vi "NI-USB-8452 SPI EEPROM Programmer.vi"() -> ()   [LabVIEW 2015]
doc: "This example shows a more generalized way to use the SPI advanced API to write data. It allows the user to change the following parameters: page size, write delay, the endianness of the address bytes, and the number of bytes in an address.\n\nThe parameters will have the following effects:\n\nTarget Page Size (bytes): This places an additional constraint on the amount of bytes written. The smaller value will be used, and that number of bytes written.\nWrite Delay Between Pages (ms): This will force a mandatory delay after writing bytes to a device.\nData Address Width: This will allow the user to specify the EEPROM Data Address as either 1 or 2 bytes.\nData Address Endianness: This control will change the ordering of the bytes in the EEPROM Data Address, note that this only has an effect if there are 2 bytes in the address.\n\nFor connection information see the NI-845x Hardware and Software manual and the manual for your specific SPI device."
uses:
  <vilib>/ni845x/ni845x.llb/ni845xControl.ctl
  <vilib>/ni845x/ni845x.llb/ni845xSpiScriptControl.ctl
  <vilib>/ni845x/ni845x.llb/NI-845x SPI Script Us Delay.vi
  <vilib>/ni845x/ni845x.llb/NI-845x SPI Script Ms Delay.vi
  <vilib>/ni845x/ni845x.llb/NI-845x SPI Close Script Reference.vi
  <vilib>/LAVA/UI Tools/Dialog/Dialog/Dialog/Dialog__lava_lib_ui_tools.lvclass
  <resource>/objmgr/NI845x.rc
panel:
  in  "Verbose?":bool
  in  "Device Data":T1(tab)
  in  "EEPROM Program Data":string[][](table)
  out "Data Bytes Written":u8[](array[numeric]) format="%x"
  out "Read Data":u8[](array[numeric]) format="%x"
  out "Hex Table":string[][](table)
  out "Bin Table":string[][](table)
  in  "EEPROM Device Type":T2(ring)
  in  "Device Mode":enum16{"SPI", "I2C", "DIO"}(ring)
  in  "CS Idle Level":enum16{"Low (Assert High)", "High (Assert Low)"}(ring)
  in  "CLK Phase (CPHS)":i32(ring) items=["0 (First Edge)", "1 (Second Edge)"]
  in  "CLK Polarity (CPOL)":i32(ring) items=["0 (Idle Low)", "1 (Idle High)"]
  in  "IO Level (V)":i32(ring)=33 items=["3.3V"=33, "2.5V"=25, "1.8V"=18, "1.5V"=15, "1.2V"=12]
  in  "CS/SS":u32
  in  "NI845x Device ID":T3="NI-8452"
  in  "CLK Rate (kHz)":u16=2000
  in  "Config INI Save":bool
  in  "Help":bool
  in  "QUIT":bool
  in  "Data Width":enum16{"8 bits", "16 bits"}(ring)
  in  "Address Width":enum16{"8 bits", "16 bits"}(ring)
  in  "Bit Pattern (Write All)":T4(ring)=enum."0xAA (0b10101010)"
  in  "Data Address Endianness":bool=TRUE
  in  "Page Write Delay (ms)":u8=3
  in  "Target Page Size (bytes)":i32=2 min=2 step=2 format="%04x"
  in  "EEPROM Data Address":u16 format="%04x"
  in  "Number of Bytes (Read)":i16=2048 min=4 step=4 format="%04x"
  in  "WRAL":u8=17 format="%08b"
  in  "ERAL":u8=18 format="%08b"
  in  "EWEN":u8=19 format="%08b"
  in  "READ":u8=6 format="%08b"
  in  "WRITE":u8=5 format="%08b"
  in  "EWDS":u8=16 format="%08b"
  in  "Write ALL Device":bool
  in  "Erase ALL Device":bool
  in  "Read Device":bool
  in  "Program Device":bool
  in  "SPI Script Reference":T5
  # "NI-USB-8452 SPI/I2C EEPROM Programmer\n(for 8, 16, 32, 64-bit Devices)"
  # "NI-8451 Device Configuration"
  # "Slave Device Configuration"
  # "Device Data"
  # "1.0_06012020"
  # "Big Endian"
  # "Little Endian"
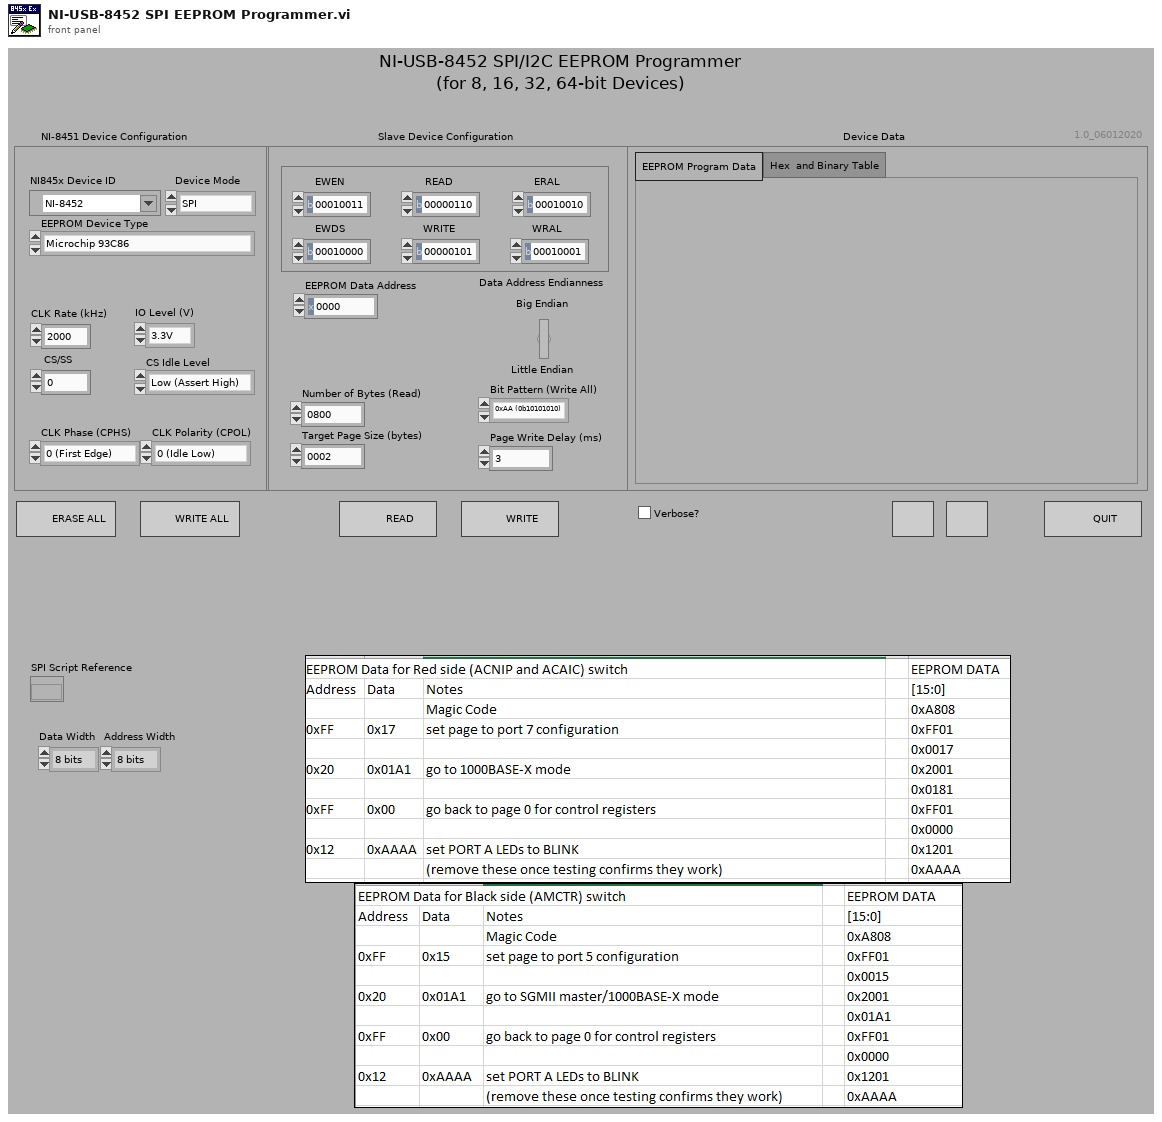
[diagram p1: front panel]
types:
  T1 = enum32{"EEPROM Program Data", "Hex  and Binary Table"}
  T2 = enum16{"Microchip 93C86", "Microchip LC56BT", "Generic EEPROM"}
  T3 = typedef "ni845xControl.ctl" = refnum<k21>
  T4 = enum8{"0xEE (0b11101110)", "0xAA (0b10101010)", "0x55 (0b01010101)", "All ONES", "All ZEROES"}
  T5 = typedef "ni845xSpiScriptControl.ctl" = refnum<k20>
  T6 = enum32{"Invalid", "Standard", "Closed", "Hidden", "Minimized", "Maximized"}
  T7 = enum32{"invalid app kind", "Development System", "Run Time System", "Student Edition", "Embedded LabVIEW", "Evaluation", "Custom"}
  T8 = cluster{"INI Path":path, "SPI Script Reference":T5, "NI845x Device ID":T3, "Device Mode":enum16{"SPI", "I2C", "DIO"}, "EEPROM Device Type":enum16{"Microchip 93C86", "Microchip LC56BT", "Generic EEPROM"}, "Core":cluster{"Current VI Reference":refnum<vi>, "Close Panel on Exit?":bool}, "IO Level (V)":i32, "CS/SS":u32, "CLK Rate (kHz)":u16, "CLK Polarity (CPOL)":i32, "CLK Phase (CPHS)":i32, " Address Width":enum16{"8 bits", "16 bits"}, "Data Width":enum16{"8 bits", "16 bits"}, "EEPROM Data Address":u16, "Number of Bytes (Read)":i16, "Target Page Size (bytes)":i32, "Page Write Delay (ms)":u8, "Array of Write Cluster Information":cluster{"EEPROM Address":u16, "Length":u32, "Data Index":u32}[], "CS Idle Level":enum16{"Low (Assert High)", "High (Assert Low)"}, "script read index":u32, "Bit Pattern (Write All)":enum8{"0xEE (0b11101110)", "0xAA (0b10101010)", "0x55 (0b01010101)", "All ONES", "All ZEROES"}, "READ":u8, "WRITE":u8, "EWEN":u8, "EWDS":u8, "WRAL":u8, "ERAL":u8, "Hex Table":string[][], "Bin Table ":string[][], "EEPROM Program Data ":string[][], "Read Data":u8[], "Data Bytes Written":u8[], "Data Address Endianness":bool, "Verbose?":bool}
  T9 = cluster{"Current VI Reference":refnum<vi>, "Close Panel on Exit?":bool}
  T10 = cluster{"EEPROM Address":u16, "Length":u32, "Data Index":u32}[]
  T11 = typedef "imagedata.ctl" = cluster{"image type":i32, "image depth":i32, "image":u8[], "mask":u8[], "colors":u32[], "Rectangle":cluster{"left":i16, "top":i16, "right":i16, "bottom":i16}}
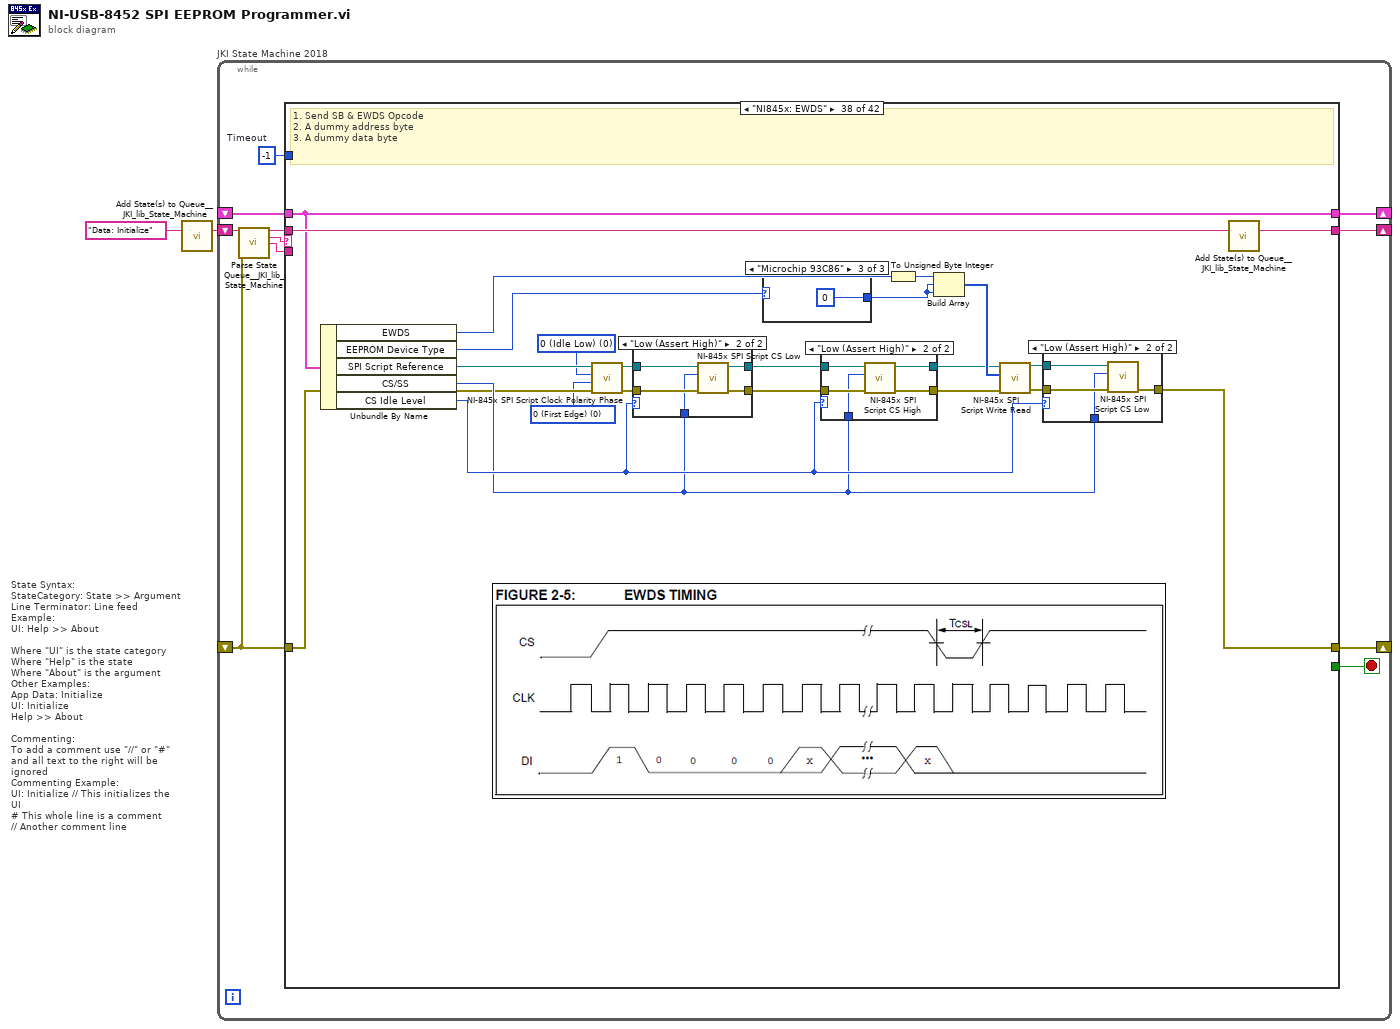
[diagram p0: block diagram]
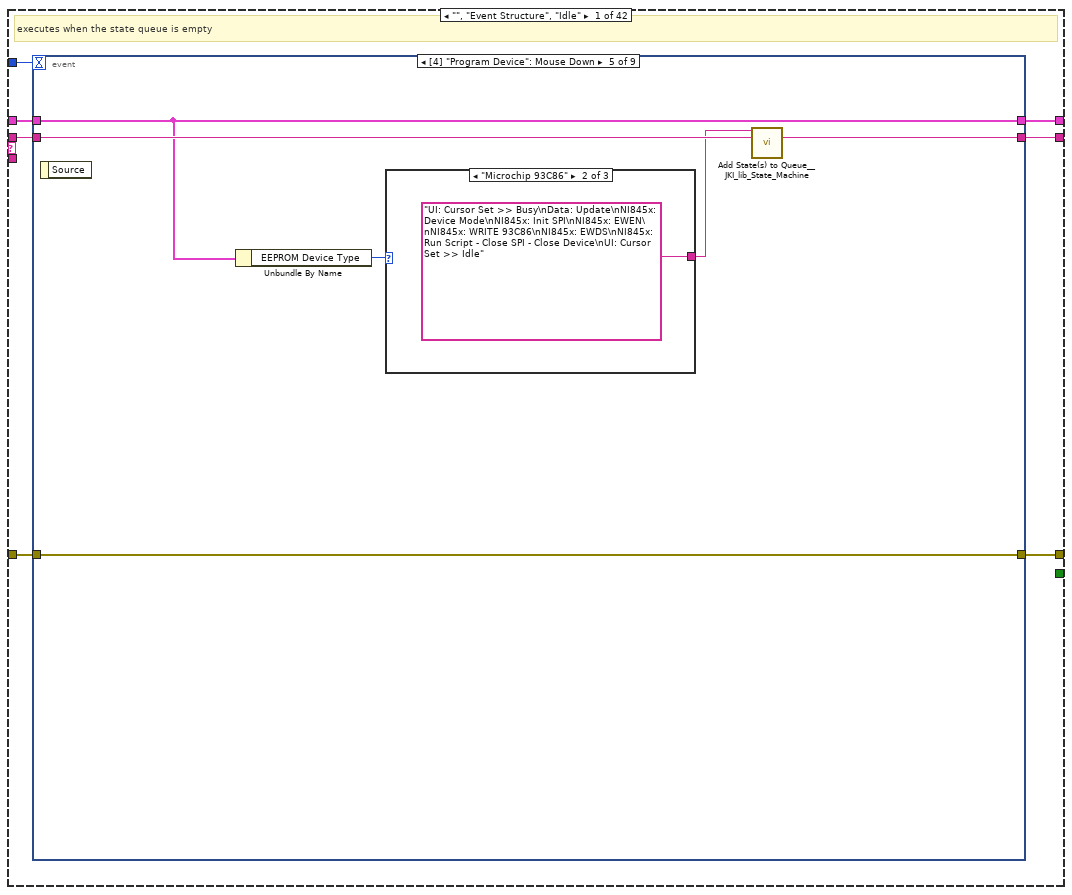
[diagram p2: hidden frame]
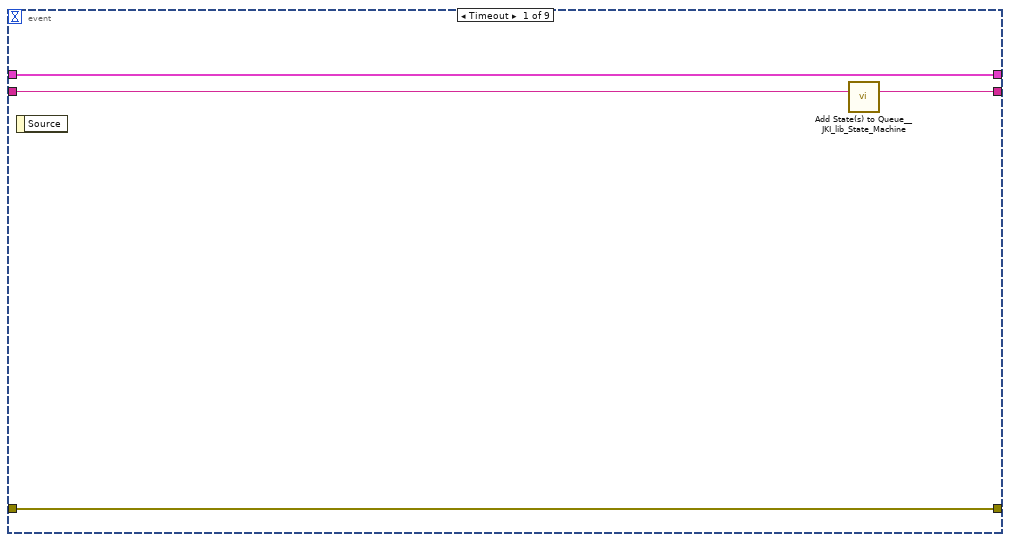
[diagram p3: hidden frame]
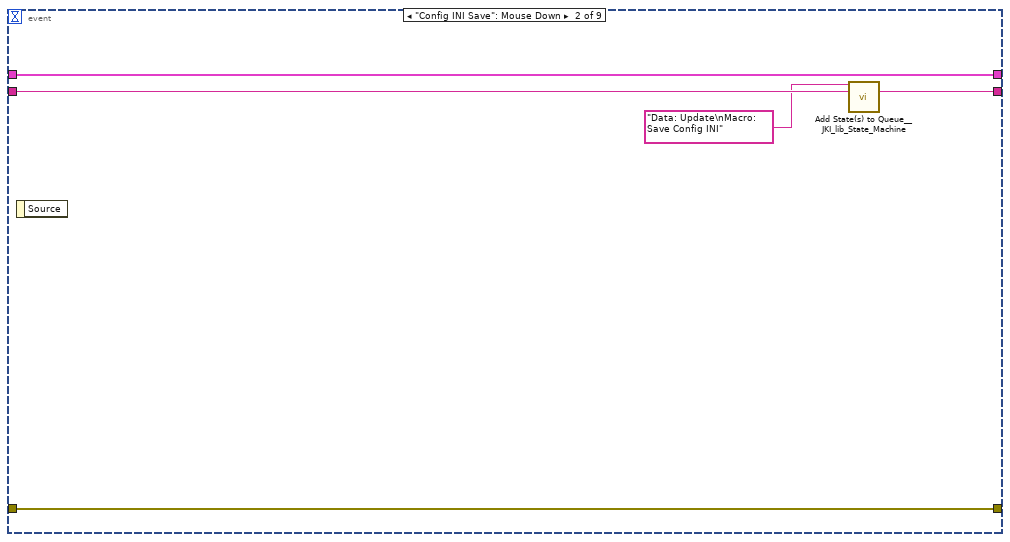
[diagram p4: hidden frame]
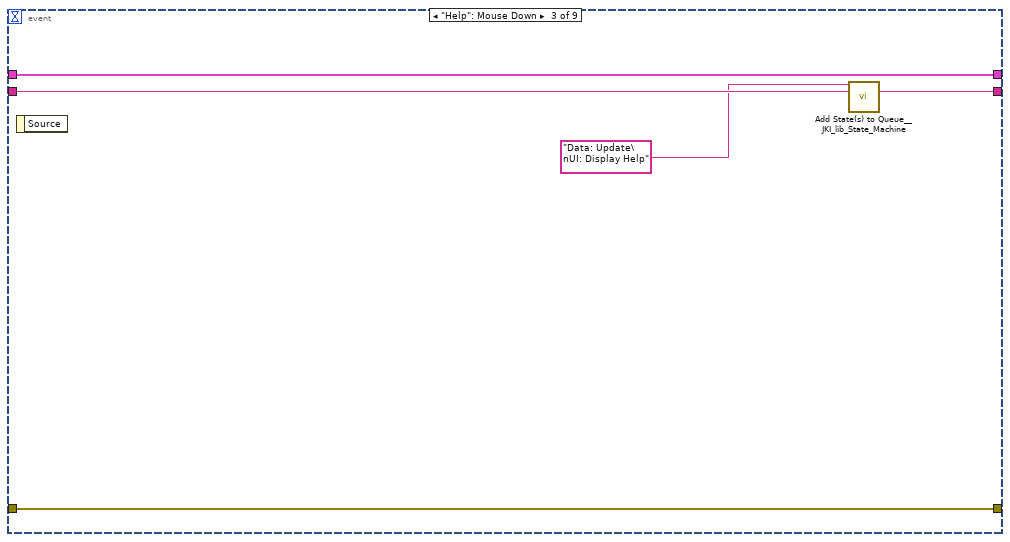
[diagram p5: hidden frame]
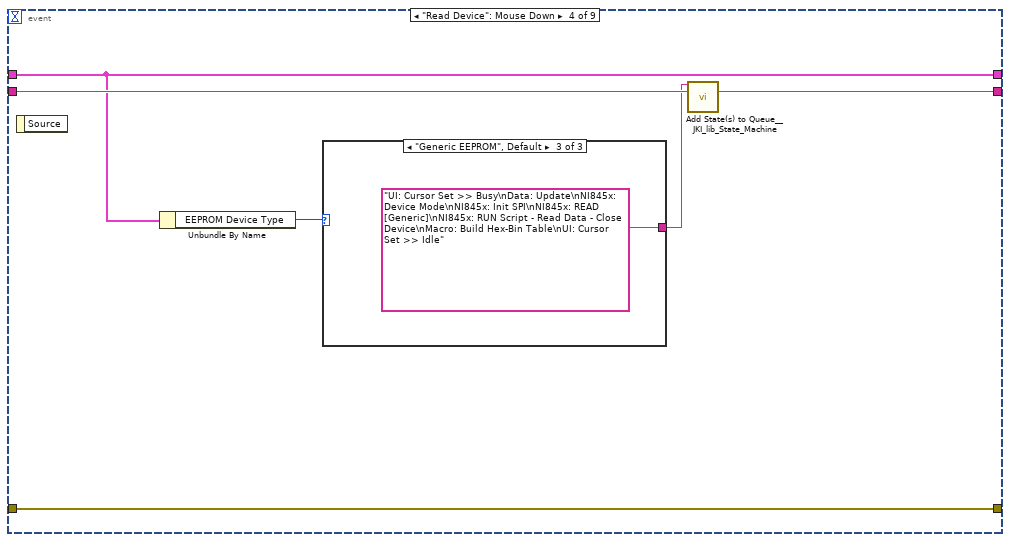
[diagram p6: hidden frame]
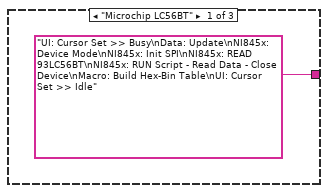
[diagram p7: hidden frame]
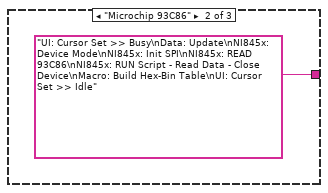
[diagram p8: hidden frame]
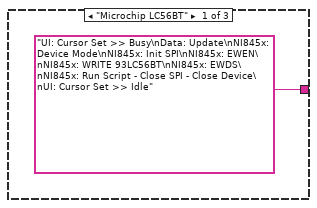
[diagram p9: hidden frame]
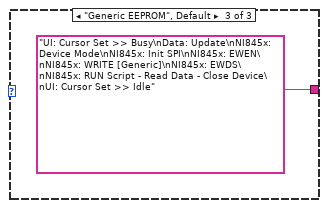
[diagram p10: hidden frame]
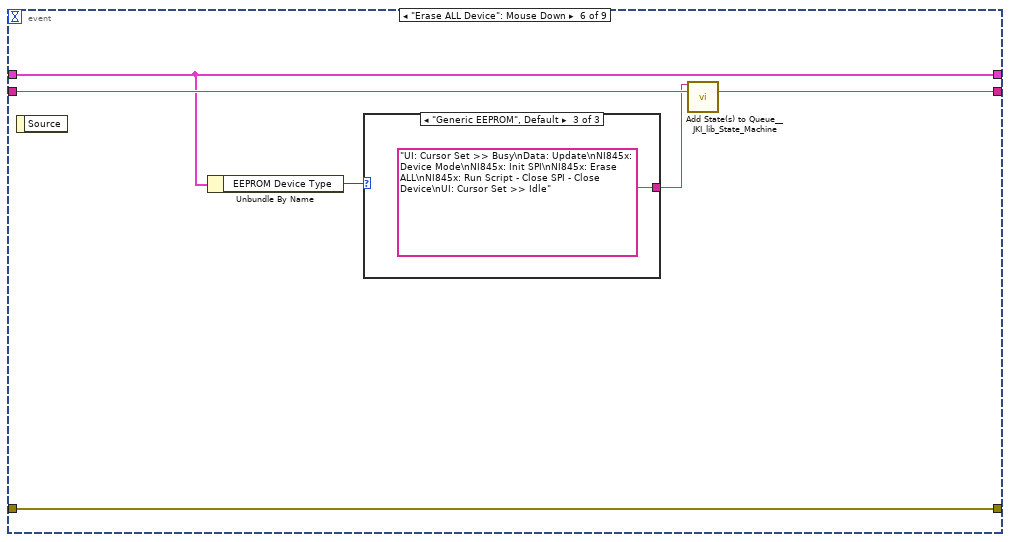
[diagram p11: hidden frame]
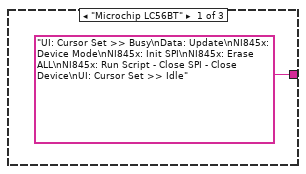
[diagram p12: hidden frame]
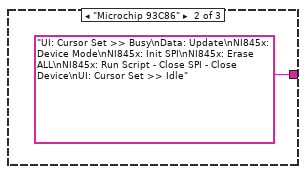
[diagram p13: hidden frame]
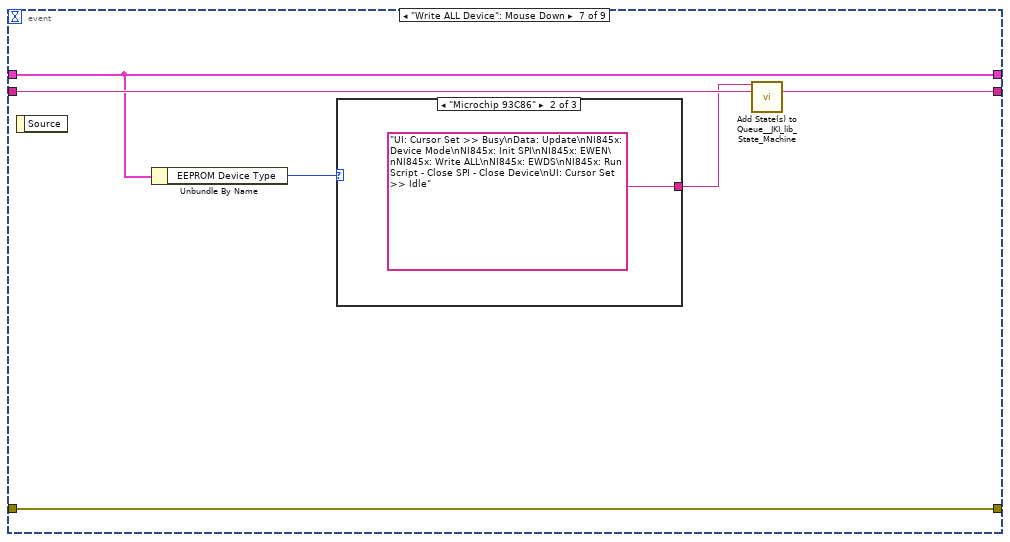
[diagram p14: hidden frame]
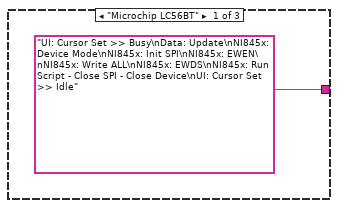
[diagram p15: hidden frame]
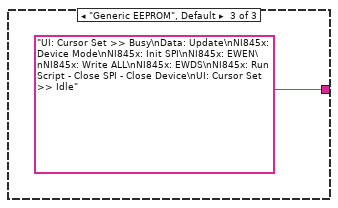
[diagram p16: hidden frame]
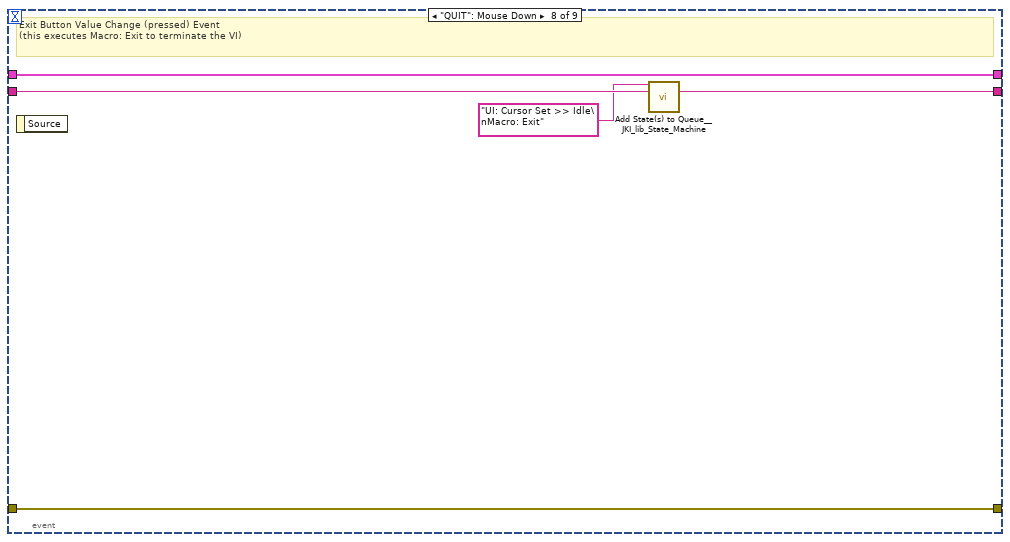
[diagram p17: hidden frame]
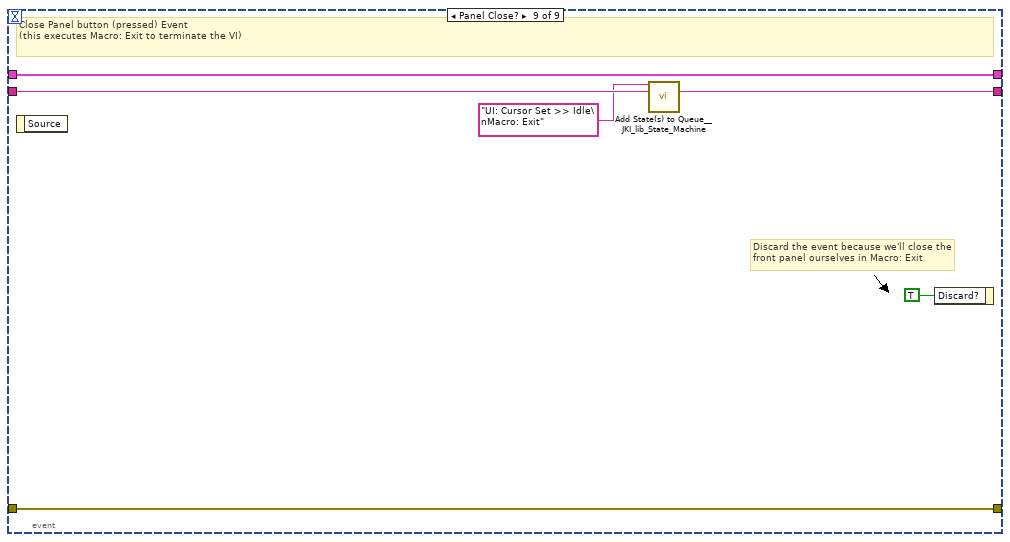
[diagram p18: hidden frame]
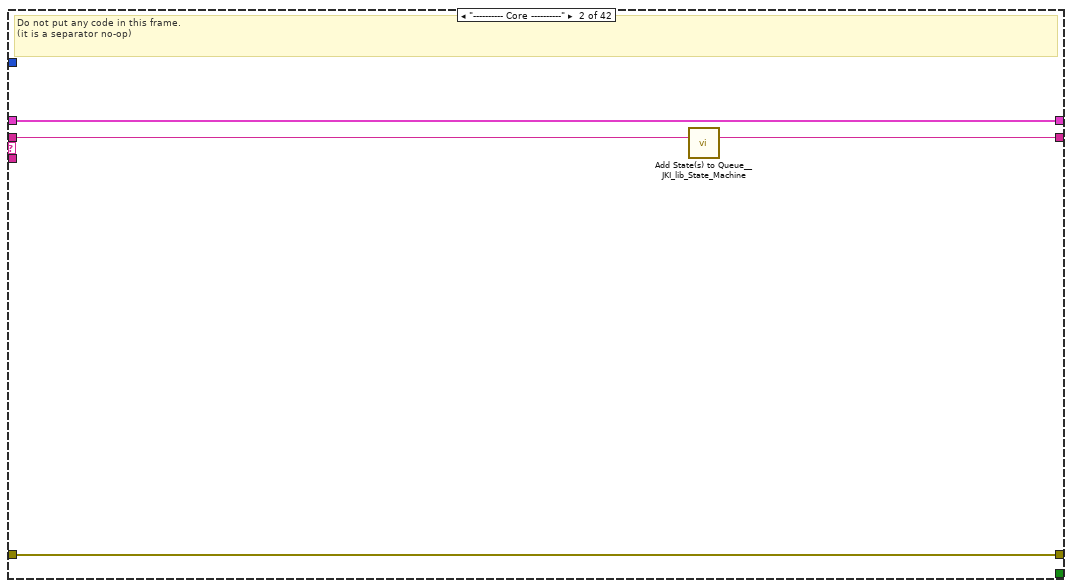
[diagram p19: hidden frame]
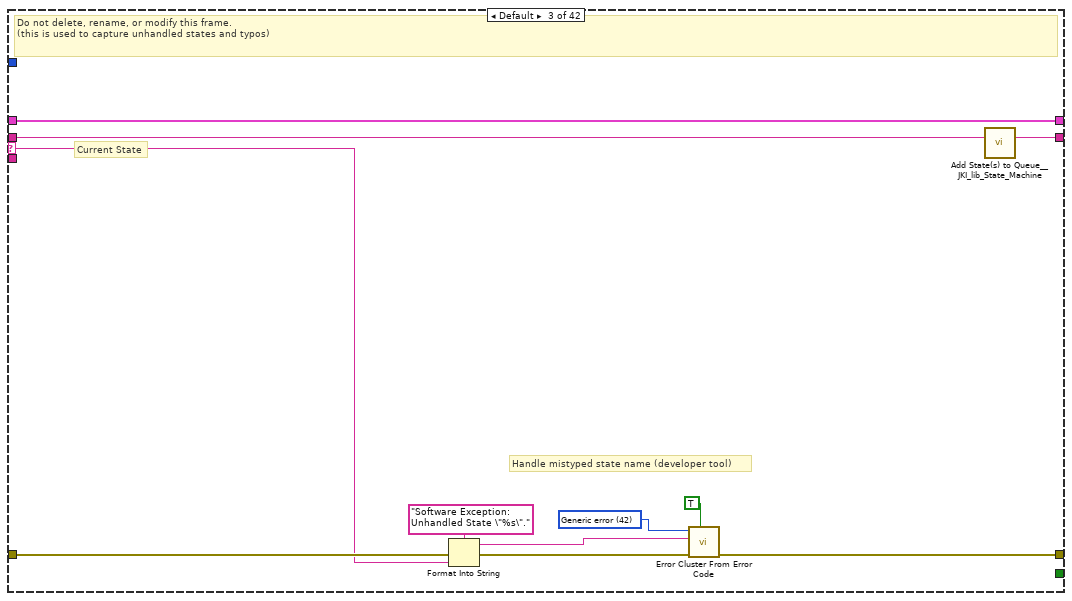
[diagram p20: hidden frame]
diagram:
  # "State Syntax:\nStateCategory: State >> Argument\nLine Terminator: Line feed\nExample:\nUI: Help >> About\n\nWhere \"UI\" is the state category\nWhere \"Help\" is the state\nWhere \"About\" is the argument\nOther Examples:\nApp Data: Initialize\nUI: Initialize\nHelp >> About\n\nCommenting:\nTo add a comment use \"//\" or \"#\" and all text to the right will be ignored\nCommenting Example:\nUI: Initialize // This initializes the UI\n# This whole line is a comment\n// Another comment line"
  n1 = call <vilib>:"Add State(s) to Queue__JKI_lib_State_Machine.vi"("State(s) in (\"\")"="Data: Initialize") -> ("States Out"=w2:string)  [unwired: 14 in]
  n2 = while "JKI State Machine 2018" {
    shift-right: [w6] -> _
    shift-left: _ -> [w5]
    shift-right: [w9] -> _
    shift-left: _ -> [w3]
    shift-right: [w8] -> _
    shift-left: w2 -> [w10]
    stop <- w7 stop-if-true
    w4 = -1  # Timeout
    n3 = call <vilib>:"Parse State Queue__JKI_lib_State_Machine.vi"("State Queue"=w10, "Error In (no error)"=w3) -> ("Remaining States"=w12:string, "Current State"=w13:string, "Arguments"=w11:string)  [unwired: 11 in]
    n4 = case shown="\"NI845x: EWDS\"" w13 {
      selector: w13 -> [_ _ w86 _ _ _ _ _ _ _ _ _ _ _ _ _ _ _ _ _ _ _ _ _ _ _ _ _ _ _ _ _ _ _ _ _ _ _ _ _ _ _]
      tunnel: w12 -> [w20 w85 w90 w109 w115 w120 w124 w169 w194 w200 w204 w208 w214 w225 w300 w308 w345 w367 w377 w390 w439 w487 w499 w511 w515 w518 w521 w525 w527 w558 w580 w630 w663 w730 w743 w812 w896 w998 w1054 w1096 w1148 w1161]
      tunnel: w11 -> [_ _ _ _ _ _ _ _ _ _ _ _ w209 w219 _ w304 _ _ _ _ _ _ _ _ _ _ _ _ _ _ _ _ _ _ _ _ _ _ _ _ _ _]
      tunnel: w5 -> [w18 w82 w88 w102 w112 w118 w121 _ w173 w195 w201 w206 w212 w221 w298 w302 w342 w365 w374 w387 w436 w480 w493 w502 w512 w516 w519 w522 w529 w548 w571 w622 w661 w725 w740 w808 w893 w991 w1048 w1091 w1141 w1154]
      tunnel: [w17 w83 w92 w106 errorcluster {"status"=FALSE, "code"=0, "source"=""} ("error out") w117 w122 w134 w192 w196 w202 w205 w210 w222 w297 w306 w343 w352 w375 w388 w437 w476 w496 w505 w513 w517 w520 w523 w530 w538 w572 w613 w651 w712 w734 w806 w886 w992 w1031 w1079 w1143 w1156] -> w9
      tunnel: w3 -> [w16 w83 w91 w106 w111 w117 w122 w129 w192 w197 w202 w205 w211 w223 w295 w305 w343 w358 w375 w388 w437 w485 w497 w506 w513 w517 w520 w523 w530 w542 w573 w621 w658 w717 w741 w807 w894 w984 w1049 w1076 w1144 w1157]
      tunnel: [w19 w84 w89 w108 w114 w119 w123 w168 w193 w199 w203 w207 w213 w224 w299 w307 w344 w366 w376 w389 w438 w486 w498 w510 w514 w518 w521 w524 w531 w557 w579 w629 w662 w729 w742 w811 w895 w997 w1053 w1095 w1147 w1160] -> w8
      tunnel: [_ _ _ _ _ TRUE _ _ _ _ _ _ _ _ _ _ _ _ _ _ _ _ _ _ _ _ _ _ _ _ _ _ _ _ _ _ _ _ _ _ _ _] -> w7
      tunnel: [w15 w82 w88 w107 w112 w118 w121 w141 w191 w195 w201 w206 w212 w221 w298 w302 w342 w365 w374 w381 w434 w480 w493 w502 w512 w516 w519 w522 w529 w537 w571 w619 w660 w723 w738 w802 w889 w991 w1035 w1083 w1131 w1154] -> w6
      tunnel: w4 -> [w14 _ _ _ _ _ _ _ _ _ _ _ _ _ _ _ _ _ _ _ _ _ _ _ _ _ _ _ _ _ _ _ _ _ _ _ _ _ _ _ _ _]
      frame "", "Event Structure", "Idle" {
        # "executes when the state queue is empty"
        n5 = event shown="[4] \"Program Device\": Mouse Down" {
          selector: _ -> [_ _ _ _ _ _ _ _ _]
          dyn-events: _ -> [_ _ _ _ _ _ _ _ _]
          timeout: w14 -> [_ _ _ _ _ _ _ _ _]
          tunnel: w20 -> [w24 w29 w34 w39 w48 w57 w66 w75 w81]
          tunnel: [w23 w28 w33 w38 w47 w56 w65 w74 w80] -> w19
          tunnel: w18 -> [w21 w26 w31 w36 w45 w54 w63 w72 w78]
          tunnel: [w22 w27 w32 w40 w49 w58 w67 w73 w79] -> w17
          tunnel: w16 -> [w22 w27 w32 w40 w49 w58 w67 w73 w79]
          tunnel: [w21 w26 w31 w36 w45 w54 w63 w72 w78] -> w15
          event Timeout {
            n6 = event-data() -> ()  [unwired: 1 in, 1 out]
            n7 = call <vilib>:"Add State(s) to Queue__JKI_lib_State_Machine.vi"("State(s) in (\"\")"=w24) -> ("States Out"=w23:string)  [unwired: 14 in]
          }
          event "Config INI Save": Mouse Down {
            n8 = event-data() -> ()  [unwired: 1 in, 1 out]
            n9 = call <vilib>:"Add State(s) to Queue__JKI_lib_State_Machine.vi"("State(s) in Front (\"\")"="Data: Update\nMacro: Save Config INI" ("State(s) in Front (\"\")"), "State(s) in (\"\")"=w29) -> ("States Out"=w28:string)  [unwired: 13 in]
          }
          event "Help": Mouse Down {
            n10 = event-data() -> ()  [unwired: 1 in, 1 out]
            n11 = call <vilib>:"Add State(s) to Queue__JKI_lib_State_Machine.vi"("State(s) in Front (\"\")"="Data: Update\nUI: Display Help" ("State(s) in Front (\"\")"), "State(s) in (\"\")"=w34) -> ("States Out"=w33:string)  [unwired: 13 in]
          }
          event "Read Device": Mouse Down {
            n12 = event-data() -> ()  [unwired: 1 in, 1 out]
            n13 = Unbundle By Name(w36) -> ("EEPROM Device Type"=w35:T2)
            n14 = case shown="\"Generic EEPROM\", Default" w35 {
              tunnel: ["UI: Cursor Set >> Busy\nData: Update\nNI845x: Device Mode\nNI845x: Init SPI\nNI845x: READ 93LC56BT\nNI845x: RUN Script - Read Data - Close Device\nMacro: Build Hex-Bin Table\nUI: Cursor Set >> Idle" ("State(s) in Front (\"\")") "UI: Cursor Set >> Busy\nData: Update\nNI845x: Device Mode\nNI845x: Init SPI\nNI845x: READ 93C86\nNI845x: RUN Script - Read Data - Close Device\nMacro: Build Hex-Bin Table\nUI: Cursor Set >> Idle" ("State(s) in Front (\"\")") "UI: Cursor Set >> Busy\nData: Update\nNI845x: Device Mode\nNI845x: Init SPI\nNI845x: READ [Generic]\nNI845x: RUN Script - Read Data - Close Device\nMacro: Build Hex-Bin Table\nUI: Cursor Set >> Idle" ("State(s) in Front (\"\")")] -> w37
              frame "Microchip LC56BT" {
              }
              frame "Microchip 93C86" {
              }
              frame "Generic EEPROM", Default {
              }
            }
            n15 = call <vilib>:"Add State(s) to Queue__JKI_lib_State_Machine.vi"("State(s) in Front (\"\")"=w37, "State(s) in (\"\")"=w39) -> ("States Out"=w38:string)  [unwired: 13 in]
          }
          event "Program Device": Mouse Down {
            n16 = event-data() -> ()  [unwired: 1 in, 1 out]
            n17 = Unbundle By Name(w45) -> ("EEPROM Device Type"=w44:T2)
            n18 = case shown="\"Microchip 93C86\"" w44 {
              tunnel: ["UI: Cursor Set >> Busy\nData: Update\nNI845x: Device Mode\nNI845x: Init SPI\nNI845x: EWEN\nNI845x: WRITE 93LC56BT\nNI845x: EWDS\nNI845x: Run Script - Close SPI - Close Device\nUI: Cursor Set >> Idle" ("State(s) in Front (\"\")") "UI: Cursor Set >> Busy\nData: Update\nNI845x: Device Mode\nNI845x: Init SPI\nNI845x: EWEN\nNI845x: WRITE 93C86\nNI845x: EWDS\nNI845x: Run Script - Close SPI - Close Device\nUI: Cursor Set >> Idle" ("State(s) in Front (\"\")") "UI: Cursor Set >> Busy\nData: Update\nNI845x: Device Mode\nNI845x: Init SPI\nNI845x: EWEN\nNI845x: WRITE [Generic]\nNI845x: EWDS\nNI845x: RUN Script - Read Data - Close Device\nUI: Cursor Set >> Idle" ("State(s) in Front (\"\")")] -> w46
              frame "Microchip LC56BT" {
              }
              frame "Microchip 93C86" {
              }
              frame "Generic EEPROM", Default {
              }
            }
            n19 = call <vilib>:"Add State(s) to Queue__JKI_lib_State_Machine.vi"("State(s) in Front (\"\")"=w46, "State(s) in (\"\")"=w48) -> ("States Out"=w47:string)  [unwired: 13 in]
          }
          event "Erase ALL Device": Mouse Down {
            n20 = event-data() -> ()  [unwired: 1 in, 1 out]
            n21 = Unbundle By Name(w54) -> ("EEPROM Device Type"=w53:T2)
            n22 = case shown="\"Generic EEPROM\", Default" w53 {
              tunnel: ["UI: Cursor Set >> Busy\nData: Update\nNI845x: Device Mode\nNI845x: Init SPI\nNI845x: Erase ALL\nNI845x: Run Script - Close SPI - Close Device\nUI: Cursor Set >> Idle" ("State(s) in Front (\"\")") "UI: Cursor Set >> Busy\nData: Update\nNI845x: Device Mode\nNI845x: Init SPI\nNI845x: Erase ALL\nNI845x: Run Script - Close SPI - Close Device\nUI: Cursor Set >> Idle" ("State(s) in Front (\"\")") "UI: Cursor Set >> Busy\nData: Update\nNI845x: Device Mode\nNI845x: Init SPI\nNI845x: Erase ALL\nNI845x: Run Script - Close SPI - Close Device\nUI: Cursor Set >> Idle" ("State(s) in Front (\"\")")] -> w55
              frame "Microchip LC56BT" {
              }
              frame "Microchip 93C86" {
              }
              frame "Generic EEPROM", Default {
              }
            }
            n23 = call <vilib>:"Add State(s) to Queue__JKI_lib_State_Machine.vi"("State(s) in Front (\"\")"=w55, "State(s) in (\"\")"=w57) -> ("States Out"=w56:string)  [unwired: 13 in]
          }
          event "Write ALL Device": Mouse Down {
            n24 = event-data() -> ()  [unwired: 1 in, 1 out]
            n25 = Unbundle By Name(w63) -> ("EEPROM Device Type"=w62:T2)
            n26 = case shown="\"Microchip 93C86\"" w62 {
              tunnel: ["UI: Cursor Set >> Busy\nData: Update\nNI845x: Device Mode\nNI845x: Init SPI\nNI845x: EWEN\nNI845x: Write ALL\nNI845x: EWDS\nNI845x: Run Script - Close SPI - Close Device\nUI: Cursor Set >> Idle" ("State(s) in Front (\"\")") "UI: Cursor Set >> Busy\nData: Update\nNI845x: Device Mode\nNI845x: Init SPI\nNI845x: EWEN\nNI845x: Write ALL\nNI845x: EWDS\nNI845x: Run Script - Close SPI - Close Device\nUI: Cursor Set >> Idle" ("State(s) in Front (\"\")") "UI: Cursor Set >> Busy\nData: Update\nNI845x: Device Mode\nNI845x: Init SPI\nNI845x: EWEN\nNI845x: Write ALL\nNI845x: EWDS\nNI845x: Run Script - Close SPI - Close Device\nUI: Cursor Set >> Idle" ("State(s) in Front (\"\")")] -> w64
              frame "Microchip LC56BT" {
              }
              frame "Microchip 93C86" {
              }
              frame "Generic EEPROM", Default {
              }
            }
            n27 = call <vilib>:"Add State(s) to Queue__JKI_lib_State_Machine.vi"("State(s) in Front (\"\")"=w64, "State(s) in (\"\")"=w66) -> ("States Out"=w65:string)  [unwired: 13 in]
          }
          event "QUIT": Mouse Down {
            # "Exit Button Value Change (pressed) Event\n(this executes Macro: Exit to terminate the VI)"
            n28 = event-data() -> ()  [unwired: 1 in, 1 out]
            n29 = call <vilib>:"Add State(s) to Queue__JKI_lib_State_Machine.vi"("State(s) in Front (\"\")"="UI: Cursor Set >> Idle\nMacro: Exit", "State(s) in (\"\")"=w75) -> ("States Out"=w74:string)  [unwired: 13 in]
          }
          event Panel Close? {
            # "Discard the event because we'll close the front panel ourselves in Macro: Exit"
            # "Close Panel button (pressed) Event\n(this executes Macro: Exit to terminate the VI)"
            n30 = event-data() -> ()  [unwired: 1 in, 1 out]
            n31 = call <vilib>:"Add State(s) to Queue__JKI_lib_State_Machine.vi"("State(s) in Front (\"\")"="UI: Cursor Set >> Idle\nMacro: Exit", "State(s) in (\"\")"=w81) -> ("States Out"=w80:string)  [unwired: 13 in]
            n32 = event-data("Discard?"=TRUE) -> ()  [unwired: 1 in, 1 out]
          }
        }
      }
      frame "---------- Core ----------" {
        # "Do not put any code in this frame.\n(it is a separator no-op)"
        n33 = call <vilib>:"Add State(s) to Queue__JKI_lib_State_Machine.vi"("State(s) in (\"\")"=w85) -> ("States Out"=w84:string)  [unwired: 14 in]
      }
      frame Default {
        w95 = 42 items=["No error", "Argument error", "Memory is full", "Out of zone", "End of file", "File already open", "Generic file I/O error", "File not found", "File permission error", "Disk is full", "Duplicate path", "Too many files open", "System feature not enabled", "Resource file not found", "Cannot add resource", "Resource not found", "Image not found", "Image memory error", "Pen does not exist", "Config type invalid", "Config token not found", "Config parse error", "Config memory error", "Bad external code format", "Bad external code offset", "External code not present", "Null window", "Destroy window error", "Null menu", "Print aborted", "Bad print record", "Print driver error", "Windows error during printing", "Memory error during printing", "Print dialog error", "Generic print error", "Invalid device refnum", "Device not found", "Device parameter error", "Device unit error", "Cannot open device", "Device call aborted", "Generic error", "Cancelled by user", "Object ID too low", "Object ID too high", "Object not in heap", "Unknown heap", "Unknown object (invalid DefProc)", "Unknown object (DefProc not in table)", "Message out of range", "Invalid (null) method", "Unknown message", "Manager call not supported", "Bad address", "Network operation in progress", "Network operation timed out", "Connection is busy", "Network attribute not supported", "Network error", "Address in use", "System out of memory", "Connection aborted", "Connection refused", "Not connected", "Already connected", "Connection closed", "Initialization error (interapplication manager)", "Bad occurrence", "Wait on unbound occurrence handler", "Occurrence queue overflow", "Datalog type conflict", "Unused", "Unrecognized type (interapplication manager)", "Memory corrupt", "Failed to make temporary DLL", "Old CIN version", "Drag socket not found", "Failed to load drop-object", "Failed to register OLE object", "Failed to release OLE object", "Format specifier type mismatch", "Unknown format specifier", "Too few format specifiers", "Too many format specifiers", "Scan failed", "Newer CIN version", "Error converting to variant", "Runtime menu error", "Password tampered", "Variant attribute not found", "Incompatible variant data type", "Event data is not available", "Event Store is not present", "Occurrence is not found", "Event Queue is not created", "Event info is not available", "Refnum passed is NULL", "Error retrieving Class GUID", "Error retrieving CoClass GUID", "Error retrieving TypeLib GUID.", "Bad built application magic bytes.", "Specific driver is different from the specific driver associated with the Logical Name.", "There is no session opened to the class driver.", "Max Error", "MAX - Error with config objects", "MAX - Error loading configuration", "MAX - Group not supported"]
        # "Current State"
        # "Handle mistyped state name (developer tool)"
        # "Do not delete, rename, or modify this frame.\n(this is used to capture unhandled states and typos)"
        n34 = Format Into String(format string="Software Exception: Unhandled State \"%s\"." ("message"), error in=w91, w86) -> (resulting string=w94:string, error out=w93:errorcluster)  [unwired: 1 in]
        n35 = call <vilib>:"Error Cluster From Error Code.vi"("show call chain? (False)"=TRUE, "error in (no error)"=w93, "error message (\"\")"=w94, "error code (0)"=w95) -> ("error out"=w92:errorcluster)  [unwired: 5 in]
        n36 = call <vilib>:"Add State(s) to Queue__JKI_lib_State_Machine.vi"("State(s) in (\"\")"=w90) -> ("States Out"=w89:string)  [unwired: 14 in]
      }
      frame "Initialize Core Data" {
        # "originally closed?"
        # "exe?"
        # "If panel starts closed or is an EXE, then close it when we exit"
        # "Do not delete, rename, or modify this frame.\n(this is used to determine panel behavior on exit)"
        n37 = property class="VI"() -> ("FP.State"=w99:T6)  [unwired: 2 in, 2 out]
        n38 = property class="App"() -> ("App.Kind"=w105:T7)  [unwired: 2 in, 2 out]
        n39 = control-ref of="Current VI Reference"() -> (w100:refnum<vi>)
        n40 = Equal?(x=w99, y=T6."Closed" ("Front Panel Window:State")) -> (x = y?=w97:bool)
        n41 = Equal?(x=w105, y=T7."Run Time System" ("Application:Kind")) -> (x = y?=w103:bool)
        n42 = Or(x=w97, y=w103) -> (x .or. y?=w101:bool)
        n43 = Bundle By Name(cluster=w102, "Core.Current VI Reference"=w100, "Core.Close Panel on Exit?"=w101) -> (w107:T8)
        n44 = call <vilib>:"Add State(s) to Queue__JKI_lib_State_Machine.vi"("State(s) in (\"\")"=w109) -> ("States Out"=w108:string)  [unwired: 14 in]
      }
      frame "Error Handler" {
        # "Unhandled Error -- Display it"
        # "Clear error"
        # "Handle any errors here.\nYou can also output any states to clean-up after errors occur"
        n45 = call <vilib>:"General Error Handler.vi"("error in (no error)"=w111) -> ()  [unwired: 10 in, 5 out]
        n46 = call <vilib>:"Add State(s) to Queue__JKI_lib_State_Machine.vi"("State(s) in Front (\"\")"="/* Post Error States", "State(s) in (\"\")"=w115) -> ("States Out"=w114:string)  [unwired: 13 in]
      }
      frame "Exit" {
        # "Do not put any code in this frame.\n(No errors that occur here will be handled.)"
        n47 = call <vilib>:"Add State(s) to Queue__JKI_lib_State_Machine.vi"("State(s) in (\"\")"=w120) -> ("States Out"=w119:string)  [unwired: 14 in]
      }
      frame "---------- Data ----------" {
        # "Do not put any code in this frame.\n(It is a separator no-op. You can make a copy of this frame to create a new Data frame)"
        n48 = call <vilib>:"Add State(s) to Queue__JKI_lib_State_Machine.vi"("State(s) in (\"\")"=w124) -> ("States Out"=w123:string)  [unwired: 14 in]
      }
      frame "Data: Initialize" {
        w125 = string[][] []  # Bin Table
        w126 = string[][] []  # Hex Table
        w128 = string[][] []  # Hex Table
        w131 = u8[] []  # Data Bytes Written
        w132 = u8[] []  # Read Data
        w142 = path ""  # INI Path
        w152 = u8[] [] ("Read Data")
        w157 = u32 0  # script read index
        w137 = T9 {"Current VI Reference"=refnum, "Close Panel on Exit?"=FALSE}  # Core
        # "do not delete - used by framework"
        # "Initialize variables & master cluster here\n(data names are defined by what you wire into the bundle function)"
        n49 = call "CreateWriteCluster.vi"("Page Size in Bytes"="Target Page Size (bytes)", "EEPROM Starting Address"="EEPROM Data Address", "Number of Bytes to Write"="Number of Bytes (Read)") -> ("Array of Write Cluster Information"=w145:T10)  [unwired: 1 in]
        n50 = control-ref of="This VI"() -> (w135:refnum<vi>)
        n51 = call "Set Config INI PATH.vi"("error in (no error)"=w129, "reference"=w135) -> ("error out"=w134:errorcluster, "appended path"=w133:path)  [unwired: 2 in]
        n52 = Bundle("INI Path"=w142, "SPI Script Reference"="SPI Script Reference", "NI845x Device ID"="NI845x Device ID", "Device Mode"="Device Mode", "EEPROM Device Type"="EEPROM Device Type", "Core"=w137, "IO Level (V)"="IO Level (V)", "CS/SS"="CS/SS", "CLK Rate (kHz)"="CLK Rate (kHz)", "CLK Polarity (CPOL)"="CLK Polarity (CPOL)", "CLK Phase (CPHS)"="CLK Phase (CPHS)", "Address Width"="Address Width", "Data Width"="Data Width", "EEPROM Data Address"="EEPROM Data Address", "Number of Bytes (Read)"="Number of Bytes (Read)", "Target Page Size (bytes)"="Target Page Size (bytes)", "Page Write Delay (ms)"="Page Write Delay (ms)", "Array of Write Cluster Information"=w145, "CS Idle Level"="CS Idle Level", "script read index"=w157, "Bit Pattern (Write All)"="Bit Pattern (Write All)", "READ"="READ", "WRITE"="WRITE", "EWEN"="EWEN", "EWDS"="EWDS", "WRAL"="WRAL", "ERAL"="ERAL", "Hex Table"=w126, "Bin Table"=w125, "EEPROM Program Data"="EEPROM Program Data", "Read Data"=w132, "Data Bytes Written"=w131, "Data Address Endianness"="Data Address Endianness", "Verbose?"="Verbose?") -> (w167:T8)  [unwired: 1 in]
        n53 = Bundle By Name(cluster=w167, "INI Path"=w133) -> (w141:T8)
        n54 = call <vilib>:"Add State(s) to Queue__JKI_lib_State_Machine.vi"("State(s) in Front (\"\")"="Initialize Core Data\nMacro: Initialize", "State(s) in (\"\")"=w169) -> ("States Out"=w168:string)  [unwired: 13 in]
        "Read Data" <- w152
        "Data Bytes Written" <- w152
        "Hex Table" <- w128
        "Bin Table" <- w128
      }
      frame "Data: Update" {
        # "Update the master cluster for any config changes"
        n55 = Unbundle By Name(w173) -> ("Hex Table"=w172:string[][], "Bin Table"=w171:string[][])
        n56 = local write "Hex Table"(w172) -> ()
        n57 = local write "Bin Table"(w171) -> ()
        n58 = local read "Number of Bytes (Read)"() -> (w186:i16)
        n59 = local read "Data Address Endianness"() -> (w175:bool)
        n60 = local read "Target Page Size (bytes)"() -> (w184:i32)
        n61 = local read "EEPROM Program Data"() -> (w170:string[][])
        n62 = local read "EEPROM Data Address"() -> (w185:u16)
        n63 = local read "Page Write Delay (ms)"() -> (w190:u8)
        n64 = local read "EEPROM Device Type"() -> (w176:T2)
        n65 = local read "NI845x Device ID"() -> (w179:T3)
        n66 = local read "Bit Pattern (Write All)"() -> (w183:T4)
        n67 = local read "Address Width"() -> (w188:enum16{"8 bits", "16 bits"})
        n68 = local read "CLK Rate (kHz)"() -> (w182:u16)
        n69 = local read "Device Mode"() -> (w178:enum16{"SPI", "I2C", "DIO"})
        n70 = local read "CS Idle Level"() -> (w189:enum16{"Low (Assert High)", "High (Assert Low)"})
        n71 = local read "IO Level (V)"() -> (w180:i32)
        n72 = local read "Data Width"() -> (w177:enum16{"8 bits", "16 bits"})
        n73 = local read "Verbose?"() -> (w174:bool)
        n74 = local read "CS/SS"() -> (w181:u32)
        n75 = call "CreateWriteCluster.vi"("Page Size in Bytes"=w184, "EEPROM Starting Address"=w185, "Number of Bytes to Write"=w186) -> ("Array of Write Cluster Information"=w187:T10)  [unwired: 1 in]
        n76 = Bundle By Name(cluster=w173, "EEPROM Device Type"=w176, "NI845x Device ID"=w179, "Device Mode"=w178, "IO Level (V)"=w180, "CS/SS"=w181, "CLK Rate (kHz)"=w182, "Bit Pattern (Write All)"=w183, "Number of Bytes (Read)"=w186, "Target Page Size (bytes)"=w184, "Page Write Delay (ms)"=w190, "CS Idle Level"=w189, "script read index"=w188, "Data Width"=w177, "EEPROM Data Address"=w185, "Array of Write Cluster Information"=w187, "Data Address Endianness"=w175, "Verbose?"=w174, "EEPROM Program Data"=w170) -> (w191:T8)
        n77 = call <vilib>:"Add State(s) to Queue__JKI_lib_State_Machine.vi"("State(s) in (\"\")"=w194) -> ("States Out"=w193:string)  [unwired: 14 in]
      }
      frame "Data: Cleanup" {
        # "Cleanup any data and references, here.\n(this is called automatically, by the Macro: Exit)"
        n78 = Unbundle By Name(w195) -> ("Core.Current VI Reference"=w198:refnum<vi>)
        n79 = Close Reference(reference=w198, error in (no error)=w197) -> (error out=w196:errorcluster)
        n80 = call <vilib>:"Add State(s) to Queue__JKI_lib_State_Machine.vi"("State(s) in (\"\")"=w200) -> ("States Out"=w199:string)  [unwired: 14 in]
      }
      frame "---------- UI ----------" {
        # "Do not put any code in this frame.\n(It is a separator no-op. You can make a copy of this frame to create a new UI frame)"
        n81 = call <vilib>:"Add State(s) to Queue__JKI_lib_State_Machine.vi"("State(s) in (\"\")"=w204) -> ("States Out"=w203:string)  [unwired: 14 in]
      }
      frame "UI: Initialize" {
        # "Initialize the User Interface, here.\n(this is called automatically, by the Macro: Init)"
        n82 = call <vilib>:"Add State(s) to Queue__JKI_lib_State_Machine.vi"("State(s) in (\"\")"=w208) -> ("States Out"=w207:string)  [unwired: 14 in]
      }
      frame "UI: Cursor Set" {
        # "Argument"
        # "Set and Unset Cursor Busy.\n(Usage: \"UI: Cursor Set >> Busy|Idle\")"
        n83 = case shown="\"Busy\"" w209 {
          tunnel: w211 -> [w216 w218]
          tunnel: [w215 w217] -> w210
          frame "Idle", Default {
            n84 = call <vilib>:"Unset Busy.vi"("error in (no error)"=w216) -> ("error out"=w215:errorcluster)  [unwired: 10 in]
          }
          frame "Busy" {
            n85 = call <vilib>:"Set Busy.vi"("error in (no error)"=w218) -> ("error out"=w217:errorcluster)  [unwired: 9 in, 1 out]
          }
        }
        n86 = call <vilib>:"Add State(s) to Queue__JKI_lib_State_Machine.vi"("State(s) in (\"\")"=w214) -> ("States Out"=w213:string)  [unwired: 14 in]
      }
      frame "UI: Front Panel State" {
        # "Argument"
        # "Set Front Panel Open or Closed\n(Usage: \"UI: Front Panel State >> Open|Close\")"
        n87 = Unbundle By Name(w221) -> ("Core.Current VI Reference"=w220:refnum<vi>)
        n88 = case shown="\"Minimize\", \"Minimized\"" w219 {
          tunnel: w223 -> [w231 w246 w257 w270 w283]
          tunnel: [w233 w247 w259 w272 w285] -> w222
          tunnel: w220 -> [w232 w244 w258 w271 w284]
          frame "Open", "Standard", Default {
            w226 = T6."Standard" ("State")
            n89 = property class="VI"(reference=w232, error in=w231) -> (reference out=w229:refnum<vi>, error out=w230:errorcluster, "FP.State"=w228:T6)
            n90 = Not Equal?(x=w228, y=w226) -> (x != y?=w227:bool)
            n91 = case shown="True" w227 {
              tunnel: [w237 w239] -> w233
              tunnel: w230 -> [w236 w239]
              tunnel: w229 -> [w235 _]
              tunnel: w226 -> [w234 _]
              frame True {
                n92 = invoke class="VI" method="FP.Open"(reference=w235, error in=w236, "Activate"=TRUE, "State"=w234) -> (error out=w237:errorcluster)  [unwired: 1 in, 4 out]
              }
              frame False {
              }
            }
          }
          frame "Close", "Closed" {
            n93 = property class="VI"(reference=w244, error in=w246) -> (reference out=w243:refnum<vi>, error out=w245:errorcluster, "FP.State"=w241:T6)
            n94 = Not Equal?(x=w241, y=T6."Closed" ("Front Panel Window:State")) -> (x != y?=w240:bool)
            n95 = case shown="True" w240 {
              tunnel: [w248 w251] -> w247
              tunnel: w245 -> [w248 w250]
              tunnel: w243 -> [_ w249]
              frame False {
              }
              frame True {
                n96 = invoke class="VI" method="FP.Close"(reference=w249, error in=w250) -> (error out=w251:errorcluster)  [unwired: 1 in, 2 out]
              }
            }
          }
          frame "Hidden", "Hide" {
            w252 = T6."Hidden" ("State")
            n97 = property class="VI"(reference=w258, error in=w257) -> (reference out=w255:refnum<vi>, error out=w256:errorcluster, "FP.State"=w254:T6)
            n98 = Not Equal?(x=w254, y=w252) -> (x != y?=w253:bool)
            n99 = case shown="True" w253 {
              tunnel: [w263 w264] -> w259
              tunnel: w256 -> [w262 w264]
              tunnel: w255 -> [w261 _]
              tunnel: w252 -> [w260 _]
              frame True {
                n100 = invoke class="VI" method="FP.Open"(reference=w261, error in=w262, "State"=w260) -> (error out=w263:errorcluster)  [unwired: 2 in, 4 out]
              }
              frame False {
              }
            }
          }
          frame "Minimize", "Minimized" {
            w265 = T6."Minimized" ("State")
            n101 = property class="VI"(reference=w271, error in=w270) -> (reference out=w268:refnum<vi>, error out=w269:errorcluster, "FP.State"=w267:T6)
            n102 = Not Equal?(x=w267, y=w265) -> (x != y?=w266:bool)
            n103 = case shown="True" w266 {
              tunnel: [w276 w277] -> w272
              tunnel: w269 -> [w275 w277]
              tunnel: w268 -> [w274 _]
              tunnel: w265 -> [w273 _]
              frame True {
                n104 = invoke class="VI" method="FP.Open"(reference=w274, error in=w275, "State"=w273) -> (error out=w276:errorcluster)  [unwired: 2 in, 4 out]
              }
              frame False {
              }
            }
          }
          frame "Maximize", "Maximized" {
            w278 = T6."Maximized" ("State")
            n105 = property class="VI"(reference=w284, error in=w283) -> (reference out=w281:refnum<vi>, error out=w282:errorcluster, "FP.State"=w280:T6)
            n106 = Not Equal?(x=w280, y=w278) -> (x != y?=w279:bool)
            n107 = case shown="True" w279 {
              tunnel: [w289 w290] -> w285
              tunnel: w282 -> [w288 w290]
              tunnel: w281 -> [w287 _]
              tunnel: w278 -> [w286 _]
              frame True {
                n108 = invoke class="VI" method="FP.Open"(reference=w287, error in=w288, "State"=w286) -> (error out=w289:errorcluster)  [unwired: 2 in, 4 out]
              }
              frame False {
              }
            }
          }
        }
        n109 = call <vilib>:"Add State(s) to Queue__JKI_lib_State_Machine.vi"("State(s) in (\"\")"=w225) -> ("States Out"=w224:string)  [unwired: 14 in]
      }
      frame "UI: Display Help" {
        n110 = call <vilib>:"Read JPEG File.vi"("error in (no error)"=w295, "path to JPEG file"=path "C:/projects/AldrinA_Test_Apps/NI-845x I2C-SPI Programmer GUI/NI8451_J6_wiring.jpg" ("Path")) -> ("error out"=w294:errorcluster, "image data"=w293:T11)  [unwired: 7 in, 1 out]
        n111 = call <vilib>:"Draw Flattened Pixmap.vi"("image data"=w293, "picture"=picture data[5B]) -> ("new picture"=w292:picture)  [unwired: 7 in]
        n112 = call "Picture Prompt.vi"("error in (no error)"=w294, "2D Picture 2"=w292) -> ("error out"=w297:errorcluster)  [unwired: 9 in]
        n113 = call <vilib>:"Add State(s) to Queue__JKI_lib_State_Machine.vi"("State(s) in (\"\")"=w300) -> ("States Out"=w299:string)  [unwired: 14 in]
      }
      frame "UI: Display Message" {
        # "// Command Format:  \"UI: Display Message >> [Window Title] [Message] [Timeout]\""
        n114 = call <vilib>:"Trim Whitespace.vi"("string"=w304) -> ("trimmed string"=w303:string)  [unwired: 1 in]
        n115 = Unbundle By Name(w302) -> ("Verbose?"=w301:bool)
        n116 = case shown="True" w301 {
          tunnel: [w309 w318] -> w306
          tunnel: w305 -> [w309 w317]
          tunnel: w303 -> [_ w316]
          frame False {
          }
          frame True {
            n117 = Empty String/Path?(string/path=w316) -> (empty?=w310:bool)
            n118 = case shown="False" w310 {
              tunnel: w316 -> [w329 _]
              tunnel: [w326 w330] -> w313
              tunnel: [w325 w330] -> w312
              tunnel: [w319 -1] -> w311
              frame False {
                w322 = string[] ["[", "]"] ("delimiters (\\s,\\t,\\r,\\n)")
                n119 = Scan String For Tokens(6:w322, 9:w329) -> (1:w326:string, 2:w328:i32, 3:w327:string)  [unwired: 4 in, 1 out]
                n120 = Scan String For Tokens(6:w322, 8:w328, 9:w327) -> (1:w325:string, 2:w323:i32, 3:w324:string)  [unwired: 3 in, 1 out]
                n121 = Scan String For Tokens(6:w322, 8:w323, 9:w324) -> (1:w321:string)  [unwired: 3 in, 3 out]
                n122 = Decimal String To Number(string=w321, default (0L)=10000 ("Timeout (-1)")) -> (number=w319:i32)  [unwired: 1 in, 1 out]
              }
              frame True {
                w330 = "Important Message" ("token string")
              }
            }
            n123 = call <vilib>:"Init Dialog__lava_lib_ui_tools.vi"("error in (no error)"=w317, "Timeout (-1)"=w311, "Message"=w312, "Dialog Title"=w313) -> ("error out"=w314:errorcluster, "Dialog out"=w315:refnum<class "Dialog__lava_lib_ui_tools.lvclass">)  [unwired: 6 in]
            n124 = while {
              tunnel: w315 -> [w339]
              shift-right: [w337] -> w318
              shift-left: w314 -> [w338]
              stop <- w334 stop-if-true
              n125 = call-dynamic "Dialog Box__lava_lib_ui_tools.vi"("error in (no error)"=w338, "Dialog in"=w339) -> ("error out"=w337:errorcluster, "timed out?"=w333:bool, "Selection"=w336:string)  [unwired: 6 in, 1 out]
              n126 = case shown="\"False\", Default" w336 {
                tunnel: [TRUE FALSE] -> w335
                frame "False", Default {
                }
                frame "True" {
                }
              }
              n127 = Or(x=w335, y=w333) -> (x .or. y?=w334:bool)
              n128 = Wait (ms)(milliseconds to wait=u32 100) -> ()  [unwired: 1 out]
            }
          }
        }
        n129 = call <vilib>:"Add State(s) to Queue__JKI_lib_State_Machine.vi"("State(s) in (\"\")"=w308) -> ("States Out"=w307:string)  [unwired: 14 in]
      }
      frame "---------- Macro ----------" {
        # "Do not put any code in this frame.\n(It is a separator no-op. You can make a copy of this frame to create a new Macro frame)"
        n130 = call <vilib>:"Add State(s) to Queue__JKI_lib_State_Machine.vi"("State(s) in (\"\")"=w345) -> ("States Out"=w344:string)  [unwired: 14 in]
      }
      frame "Macro: Initialize" {
        w349 = string[][] [] ("Hex Table")
        w355 = string[] ["Address", "1", "2", "3", "4"] ("Column Header Strings[]")
        w351 = FALSE ("QUIT")
        w364 = "UI: Initialize\nUI: Front Panel State >> Open\nMacro: Load Config INI\nData: Update"  # UI: Initialize UI: Front Panel State >> Open Macro: Load Config INI Data: Update
        # "Initialization Macro\n(This is called once, when the VI starts)"
        n131 = property on="Hex Table" class="Tbl (strict)"(error in=w358, "Column Headers[]"=w355, "Number of Columns"=u32 5, "Value"=w349) -> (error out=w356:errorcluster)  [unwired: 1 in, 1 out]
        n132 = property on="Bin Table" class="Tbl (strict)"(error in=w356, "Column Headers[]"=w355, "Number of Columns"=u32 5, "Value"=w349) -> (error out=w350:errorcluster)  [unwired: 1 in, 1 out]
        n133 = property on="EEPROM Program Data" class="Tbl (strict)"(error in=w350, "Column Headers[]"=string[] ["Address", "Data"] ("Column Header Strings[]"), "Number of Columns"=u32 2, "Value"=w349) -> (error out=w346:errorcluster)  [unwired: 1 in, 1 out]
        n134 = property on="QUIT" class="Bool (strict)"(error in=w346, "Value"=w351) -> (error out=w360:errorcluster)  [unwired: 1 in, 1 out]
        n135 = property on="Read Device" class="Bool (strict)"(error in=w360, "Value"=w351) -> (error out=w361:errorcluster)  [unwired: 1 in, 1 out]
        n136 = property on="Program Device" class="Bool (strict)"(error in=w361, "Value"=w351) -> (error out=w362:errorcluster)  [unwired: 1 in, 1 out]
        n137 = property on="Write ALL Device" class="Bool (strict)"(error in=w362, "Value"=w351) -> (error out=w363:errorcluster)  [unwired: 1 in, 1 out]
        n138 = property on="Erase ALL Device" class="Bool (strict)"(error in=w363, "Value"=w351) -> (error out=w359:errorcluster)  [unwired: 1 in, 1 out]
        n139 = property on="Help" class="Bool (strict)"(error in=w359, "Value"=w351) -> (error out=w353:errorcluster)  [unwired: 1 in, 1 out]
        n140 = property on="Config INI Save" class="Bool (strict)"(error in=w353, "Value"=w351) -> (error out=w352:errorcluster)  [unwired: 1 in, 1 out]
        n141 = call <vilib>:"Add State(s) to Queue__JKI_lib_State_Machine.vi"("State(s) in Front (\"\")"=w364, "State(s) in (\"\")"=w367) -> ("States Out"=w366:string)  [unwired: 13 in]
      }
      frame "Macro: Exit" {
        # "Exit Macro\n(This is called once, when the VI exits)"
        n142 = Unbundle By Name(w374) -> ("Core.Close Panel on Exit?"=w373:bool)
        n143 = Select(t="UI: Front Panel State >> Close", s=w373, f="") -> (s? t:f=w370:string)
        n144 = call <vilib>:"Add State(s) to Queue__JKI_lib_State_Machine.vi"("State(s) in (\"\")"=w370, "State(s) at Back (\"\")"="Data: Cleanup\nMacro: Save Config INI\nExit") -> ("States Out"=w368:string)  [unwired: 13 in]
        n145 = call <vilib>:"Add State(s) to Queue__JKI_lib_State_Machine.vi"("State(s) in Front (\"\")"=w368, "State(s) in (\"\")"=w377) -> ("States Out"=w376:string)  [unwired: 13 in]
      }
      frame "Macro: Build Hex-Bin Table [SAVE]" {
        w382 = string[][] [] ("array")
        # "Update the Hex strings display post data capture from device"
        n146 = Unbundle By Name(w387) -> ("Read Data"=w386:u8[])
        n147 = Array Size(array=w386) -> (size(s)=w385:i32)
        n148 = Quotient & Remainder(x=w385, y=4) -> (floor(x/y)=w383:i32)  [unwired: 1 out]
        n149 = for {
          N: w383 -> [_]
          shift-right: [w409] -> _
          shift-left: w386 -> [w408]
          shift-right: [w404] -> w379
          shift-left: w382 -> [w403]
          shift-right: [w392] -> w380
          shift-left: w382 -> [w391]
          i -> [w394]
          (unwired) string[] [] ("array")
          w405 = 4 ("length")
          (unwired) ""
          # "Extract 4 bytes at a time.\nRemaining elements to shift register"
          n150 = Delete From Array(array=w408, length=w405) -> (deleted portion=w410:u8[], array with subset deleted=w409:u8[])  [unwired: 1 in]
          n151 = for {
            tunnel: w410 -> [w425] mode=indexing
            shift-right: [w423] -> _
            shift-left: _ -> [w422]
            shift-right: [w421] -> _
            shift-left: _ -> [w420]
            shift-right: [w417] -> w402
            shift-left: _ -> [w415]
            shift-right: [w411] -> w395
            shift-left: _ -> [w412]
            i -> [w414]
            w418 = "\t"
            n152 = Number To Hexadecimal String(2:w425) -> (0:w424:string)  [unwired: 1 in]
            n153 = call "Hex_String_to_Binary_String.vi"("bitness"=enum16{"8", "16", "32", "64"}."8", "Hexadecimal String"=w424) -> ("Hex String"=w416:string, "Binary String"=w413:string)  [unwired: 1 in, 1 out]
            n154 = Concatenate Strings(w422, w413, w418) -> (w423:string)
            n155 = Insert Into Array(array=w412, index=w414, new element=w413) -> (w411:string[])
            n156 = Concatenate Strings(w420, w416, w418) -> (w421:string)
            n157 = Insert Into Array(array=w415, index=w414, new element=w416) -> (w417:string[])
          }
          n158 = Multiply(x=w405, y=w394) -> (x*y=w406:i32)
          n159 = Number To Hexadecimal String(1:i16 4 ("width (-)"), 2:w406) -> (0:w396:string)
          n160 = Build Array (concatenate)(w396, w402) -> (w400:string[])
          n161 = Build Array (concatenate)(w396, w395) -> (w397:string[])
          n162 = Reshape Array(w400, 5 ("dimension size")) -> (w399:string[])
          n163 = Reshape Array(w397, 5 ("dimension size")) -> (w393:string[])
          n164 = Insert Into Array(array=w391, index (row)=w394, new element=w393) -> (w392:string[][])  [unwired: 1 in]
          n165 = Insert Into Array(array=w403, index (row)=w394, new element=w399) -> (w404:string[][])  [unwired: 1 in]
        }
        n166 = local write "Bin Table"(w380) -> ()
        n167 = local write "Hex Table"(w379) -> ()
        n168 = call <vilib>:"Add State(s) to Queue__JKI_lib_State_Machine.vi"("State(s) in Front (\"\")"="UI: Display Message >>  [Alert!][Hex & Binary Table Parsed][10000]" ("State(s) in Front (\"\")"), "State(s) in (\"\")"=w390) -> ("States Out"=w389:string)  [unwired: 13 in]
        n169 = Bundle By Name(cluster=w387, "Bin Table"=w380, "Hex Table"=w379) -> (w381:T8)
      }
      frame "Macro: Build Hex-Bin Table" {
        w431 = string[][] [] ("array")
        # "Update the Hex strings display post data capture from device"
        n170 = Unbundle By Name(w436) -> ("Read Data"=w432:u8[], "Target Page Size (bytes)"=w428:i32)
        n171 = Array Size(array=w432) -> (size(s)=w435:i32)
        n172 = Quotient & Remainder(x=w435, y=w428) -> (floor(x/y)=w427:i32)  [unwired: 1 out]
        n173 = Increment(x=w427) -> (x+1=w426:i32)
        n174 = for {
          N: w426 -> [_]
          shift-right: [w459] -> _
          shift-left: w432 -> [w458]
          shift-right: [w456] -> w430
          shift-left: w431 -> [w455]
          shift-right: [w447] -> w429
          shift-left: w431 -> [w446]
          tunnel: w428 -> [w442]
          i -> [w440]
          # "Extract n bytes at a time (per page size)\nRemaining elements to shift register"
          n175 = Delete From Array(array=w458, length=w442, index=0) -> (deleted portion=w460:u8[], array with subset deleted=w459:u8[])
          n176 = for {
            tunnel: w460 -> [w475] mode=indexing
            shift-right: [w473] -> _
            shift-left: "" -> [w472]
            shift-right: [w471] -> _
            shift-left: _ -> [w470]
            shift-right: [w467] -> w454
            shift-left: string[] [] ("array") -> [w465]
            shift-right: [w461] -> w449
            shift-left: _ -> [w462]
            i -> [w464]
            w468 = "\t"
            n177 = Number To Hexadecimal String(2:w475) -> (0:w474:string)  [unwired: 1 in]
            n178 = call "Hex_String_to_Binary_String.vi"("bitness"=enum16{"8", "16", "32", "64"}."8", "Hexadecimal String"=w474) -> ("Hex String"=w466:string, "Binary String"=w463:string)  [unwired: 1 in, 1 out]
            n179 = Concatenate Strings(w472, w463, w468) -> (w473:string)
            n180 = Insert Into Array(array=w462, index=w464, new element=w463) -> (w461:string[])
            n181 = Concatenate Strings(w470, w466, w468) -> (w471:string)
            n182 = Insert Into Array(array=w465, index=w464, new element=w466) -> (w467:string[])
          }
          n183 = Number To Hexadecimal String(1:i16 4 ("width (-)"), 2:w440) -> (0:w450:string)
          n184 = Increment(x=w442) -> (x+1=w441:i32)
          n185 = Build Array (concatenate)(w450, w454) -> (w453:string[])
          n186 = Build Array (concatenate)(w450, w449) -> (w451:string[])
          n187 = Reshape Array(w453, w441) -> (w452:string[])
          n188 = Reshape Array(w451, w441) -> (w448:string[])
          n189 = Insert Into Array(array=w446, index (row)=w440, new element=w448) -> (w447:string[][])  [unwired: 1 in]
          n190 = Insert Into Array(array=w455, index (row)=w440, new element=w452) -> (w456:string[][])  [unwired: 1 in]
        }
        n191 = call <vilib>:"Add State(s) to Queue__JKI_lib_State_Machine.vi"("State(s) in Front (\"\")"="UI: Display Message >>  [Alert!][Hex & Binary Table Parsed][10000]" ("State(s) in Front (\"\")"), "State(s) in (\"\")"=w439) -> ("States Out"=w438:string)  [unwired: 13 in]
        n192 = local write "Bin Table"(w429) -> ()
        n193 = local write "Hex Table"(w430) -> ()
        n194 = Bundle By Name(cluster=w436, "Bin Table"=w429, "Hex Table"=w430) -> (w434:T8)
      }
      frame "Macro: Load Binary File" {
        # "Do not put any code in this frame.\n(It is a separator no-op. You can make a copy of this frame to create a new Macro frame)"
        n195 = Unbundle By Name(w480) -> ("Data Address Endianness"=w479:bool)
        n196 = Boolean To (0,1)(Boolean=w479) -> (0, 1=w478:i16)
        n197 = call "File Dialog"("prompt"="Find and Select the Binary or Hex File to Load to EEPROM", "error in"=w485, "pattern (all files)"="*.bin;*.hex") -> ("selected path"=w482:path, "error out"=w481:errorcluster)  [unwired: 9 in, 2 out]
        n198 = Read from Binary File(5:"" ("data type"), 8:w481, 9:w478, 11:w482) -> (0:w476:errorcluster)  [unwired: 2 in, 3 out]
        n199 = call <vilib>:"Add State(s) to Queue__JKI_lib_State_Machine.vi"("State(s) in (\"\")"=w487) -> ("States Out"=w486:string)  [unwired: 14 in]
      }
      frame "Macro: Save Config INI" {
        # "// Save control values & states to INI file\n// Config.INI saved in directory as this VI"
        n200 = Unbundle By Name(w493) -> ("INI Path"=w492:path)
        n201 = control-ref of="This VI"() -> (w494:refnum<vi>)
        n202 = call "Utility Write Config INI to File.vi"("File Type"=".ini", "Error In"=w497, "reference"=w494, "Path In"=w492) -> ("Error Out"=w496:errorcluster, "Path Out"=w491:path)  [unwired: 6 in]
        n203 = Path To String(path=w491) -> (string=w489:string)
        n204 = Format Into String(format string="UI: Display Message >> [Configuration INI Saved To PATH: ][%s][10000]" ("State(s) in Front (\"\")"), w489) -> (resulting string=w488:string)  [unwired: 2 in, 1 out]
        n205 = call <vilib>:"Add State(s) to Queue__JKI_lib_State_Machine.vi"("State(s) in Front (\"\")"=w488, "State(s) in (\"\")"=w499) -> ("States Out"=w498:string)  [unwired: 13 in]
      }
      frame "Macro: Load Config INI" {
        n206 = Unbundle By Name(w502) -> ("INI Path"=w501:path)
        n207 = control-ref of="This VI"() -> (w509:refnum<vi>)
        n208 = call "Utility Load Config INI from File.vi"("File Type"=".ini", "Error In"=w506, "reference"=w509, "Path In"=w501) -> ("Error Out"=w505:errorcluster, "Path Out"=w508:path)  [unwired: 6 in]
        n209 = Path To String(path=w508) -> (string=w503:string)
        n210 = Format Into String(format string="UI: Display Message >> [Configuration INI Loaded From PATH: ][%s][10000]" ("State(s) in Front (\"\")"), w503) -> (resulting string=w500:string)  [unwired: 2 in, 1 out]
        n211 = call <vilib>:"Add State(s) to Queue__JKI_lib_State_Machine.vi"("State(s) in Front (\"\")"=w500, "State(s) in (\"\")"=w511) -> ("States Out"=w510:string)  [unwired: 13 in]
      }
      frame "---------- NI845x: Template ----------" {
        # "Template Separator\n(You can make a copy of, or modify, this frame)"
        n212 = call <vilib>:"Add State(s) to Queue__JKI_lib_State_Machine.vi"("State(s) in (\"\")"=w515) -> ("States Out"=w514:string)  [unwired: 14 in]
      }
      frame "93LC56BT Notes" {
        # "Template Separator\n(You can make a copy of, or modify, this frame)"
        n213 = disable-structure shown="Disabled" {
          frame Enabled {
          }
          frame Disabled {
          }
          frame Disabled {
          }
        }
      }
      frame "93C86 Notes" {
        # "Microchip 93C76/86 8K/16K 5.0V Microwire Serial EEPROM"
        n214 = disable-structure shown="Enabled" {
          frame Enabled {
          }
          frame Disabled {
          }
          frame Disabled {
          }
        }
      }
      frame "NI845x: Prep EEPROM Data" {
        (unwired) u16[][] [[65281, 21], [8193, 417], [65281, 0], [4609, 43690]]
        # "Template Separator\n(You can make a copy of, or modify, this frame)"
        n215 = call <vilib>:"Add State(s) to Queue__JKI_lib_State_Machine.vi"("State(s) in (\"\")"=w525) -> ("States Out"=w524:string)  [unwired: 14 in]
      }
      frame "NI845x: Device Mode" {
        # "Send Message if Mode is not yet supported\nCommand Format:  \"UI: Display Message >> [Window Title] [Message] [Timeout]\""
        n216 = Unbundle By Name(w529) -> ("Device Mode"=w528:enum16{"SPI", "I2C", "DIO"})
        n217 = case shown="\"DIO\"" w528 {
          tunnel: [w532 "UI: Display Message >>  [Alert!][I2C Mode is NOT supported at this time][10000]\n" "UI: Display Message >>  [Alert!][DIO Mode is NOT supported at this time][10000]\n"] -> w526
          tunnel: w527 -> [w532 _ _]
          frame "SPI", Default {
          }
          frame "I2C" {
          }
          frame "DIO" {
          }
        }
        n218 = call <vilib>:"Add State(s) to Queue__JKI_lib_State_Machine.vi"("State(s) in (\"\")"=w526) -> ("States Out"=w531:string)  [unwired: 14 in]
      }
      frame "NI845x: Init SPI" {
        # "The Microchip EEPROMs' CS idle\nstate is LOW and asserted HIGH\nso set SPI to LOW post INIT."
        # "Step 1: Set the I/O reference voltage:\n\nNot all NI-845x hardware support all voltage levels. \nPlease consult your hardware documentation for more information.\n\nStep 2: Create the script and configure the SPI bus:\n\na) Create the script\nb) Switch the SPI bus pins into master mode. \n    This automatically sets all CS lines to be high.\nc) Configure the Phase and Plarity to mode 0, in \n    which the polarity and phase are both set to \n    zero, however this may be configured for \n    other EEPROMs. \nd) Configure the Clock rate as set by the front \n    panel control."
        # "NI845x only supports 8-bits per sample. \nNI8452 supports 8-64 bits per sample."
        n219 = Unbundle By Name(w548) -> ("CS/SS"=w543:u32, "CLK Rate (kHz)"=w544:u16, "NI845x Device ID"=w547:T3, "IO Level (V)"=w546:i32, "CLK Polarity (CPOL)"=w541:i32, "CLK Phase (CPHS)"=w540:i32)
        n220 = property on="Property Node" class="NI-845x Device"(reference=w547, error in=w542, "IoVoltLevel"=w546) -> (error out=w552:errorcluster)  [unwired: 1 out]
        n221 = call <vilib>:"NI-845x SPI Create Script Reference.vi"("error in (no error)"=w552) -> ("error out"=w551:errorcluster, "spi script reference"=w545:T5)  [unwired: 9 out]
        n222 = call <vilib>:"NI-845x SPI Script Enable SPI.vi"("error in (no error)"=w551, "spi script reference in"=w545) -> ("error out"=w553:errorcluster, "spi script reference out"=w554:T5)  [unwired: 8 out]
        n223 = Bundle By Name(cluster=w548, "SPI Script Reference"=w545) -> (w537:T8)
        n224 = call <vilib>:"NI-845x SPI Script Clock Polarity Phase.vi"("error in (no error)"=w553, "clock phase (0)"=w540, "clock polarity (0)"=w541, "spi script reference in"=w554) -> ("error out"=w549:errorcluster, "spi script reference out"=w550:T5)  [unwired: 2 in, 4 out]
        n225 = call <vilib>:"NI-845x SPI Script Clock Rate.vi"("error in (no error)"=w549, "clock rate in kHz (1000)"=w544, "spi script reference in"=w550) -> ("error out"=w555:errorcluster, "spi script reference out"=w556:T5)  [unwired: 1 in, 6 out]
        n226 = Unbundle By Name(w537) -> ("EEPROM Device Type"=w536:T2)
        n227 = call <vilib>:"NI-845x SPI Script CS Low.vi"("error in (no error)"=w555, "chip select (0)"=w543, "spi script reference in"=w556) -> ("error out"=w539:errorcluster, "spi script reference out"=w535:T5)  [unwired: 7 in]
        n228 = case shown="\"Microchip 93C86\"" w536 {
          tunnel: w539 -> [w560 w564]
          tunnel: [w560 w563] -> w538
          tunnel: w535 -> [w559 w562]
          tunnel: [w559 w561] -> _
          frame "Microchip LC56BT", Default {
            # "NI-8451 is 8-bit ONLY"
          }
          frame "Microchip 93C86" {
            # "Change to 16 bits with NI8452"
            n229 = call <vilib>:"NI-845x SPI Script Num Bits Per Sample.vi"("error in (no error)"=w564, "num bits per sample (8)"=u16 16, "spi script reference in"=w562) -> ("error out"=w563:errorcluster, "spi script reference out"=w561:T5)  [unwired: 7 in]
          }
        }
        n230 = call <vilib>:"Add State(s) to Queue__JKI_lib_State_Machine.vi"("State(s) in (\"\")"=w558) -> ("States Out"=w557:string)  [unwired: 14 in]
      }
      frame "NI845x: EWEN" {
        # "The Microchip 93C86 CS idle\nstate is LOW and asserted HIGH"
        # "1. Send SB & EWEN Opcode for 93LC56BT\n2. A dummy address byte\n3. A dummy data byte"
        n231 = Unbundle By Name(w571) -> ("EEPROM Device Type"=w566:T2, "EWEN"=w568:u8, "SPI Script Reference"=w570:T5, "CS/SS"=w567:u32, "CS Idle Level"=w569:enum16{"Low (Assert High)", "High (Assert Low)"})
        n232 = case shown="\"Microchip LC56BT\", Default" w566 {
          tunnel: [w582 w586] -> w578
          tunnel: w568 -> [w581 w585]
          frame "Microchip LC56BT", Default {
            w583 = u8 0
            # "16-bit Data & 8-bit Address"
            n233 = Build Array(w581, w583, w583) -> (w582:u8[])
          }
          frame "Microchip 93C86" {
            w584 = u16 0
            # "16-bit Data & Address"
            n234 = Build Array(w585, w584, w584) -> (w586:u16[])
          }
        }
        n235 = case shown="\"Low (Assert High)\"" w569 {
          tunnel: [w599 w604] -> w575
          tunnel: [w598 w603] -> w574
          tunnel: w573 -> [w597 w602]
          tunnel: w570 -> [w596 w601]
          tunnel: w567 -> [w595 w600]
          frame "Low (Assert High)" {
            n236 = call <vilib>:"NI-845x SPI Script CS High.vi"("error in (no error)"=w597, "chip select (0)"=w595, "spi script reference in"=w596) -> ("error out"=w598:errorcluster, "spi script reference out"=w599:T5)  [unwired: 7 in]
          }
          frame "High (Assert Low)", Default {
            n237 = call <vilib>:"NI-845x SPI Script CS Low.vi"("error in (no error)"=w602, "chip select (0)"=w600, "spi script reference in"=w601) -> ("error out"=w603:errorcluster, "spi script reference out"=w604:T5)  [unwired: 7 in]
          }
        }
        n238 = call <vilib>:"NI-845x SPI Script Write Read.vi"("error in (no error)"=w574, "write data"=w578, "spi script reference in"=w575) -> ("error out"=w576:errorcluster, "spi script reference out"=w577:T5)  [unwired: 1 in, 6 out]
        n239 = case shown="\"Low (Assert High)\"" w569 {
          tunnel: w577 -> [w590 w594]
          tunnel: w576 -> [w589 w593]
          tunnel: [w588 w592] -> w572
          tunnel: w567 -> [w587 w591]
          frame "High (Assert Low)" {
            n240 = call <vilib>:"NI-845x SPI Script CS High.vi"("error in (no error)"=w589, "chip select (0)"=w587, "spi script reference in"=w590) -> ("error out"=w588:errorcluster)  [unwired: 7 in, 1 out]
          }
          frame "Low (Assert High)" {
            n241 = call <vilib>:"NI-845x SPI Script CS Low.vi"("error in (no error)"=w593, "chip select (0)"=w591, "spi script reference in"=w594) -> ("error out"=w592:errorcluster)  [unwired: 7 in, 1 out]
          }
        }
        n242 = call <vilib>:"Add State(s) to Queue__JKI_lib_State_Machine.vi"("State(s) in (\"\")"=w580) -> ("States Out"=w579:string)  [unwired: 14 in]
      }
      frame "NI845x: READ 93LC56BT" {
        # "For Microchip LC56BT the MSB is transmitted first (high endian)\nThe Microchip LC56BT CS idle state is LOW and asserted HIGH"
        n243 = Unbundle By Name(w622) -> ("CS/SS"=w623:u32, "CS Idle Level"=w620:enum16{"Low (Assert High)", "High (Assert Low)"}, "SPI Script Reference"=w624:T5, "READ"=w608:u8, "EEPROM Data Address"=w607:u16, "Number of Bytes (Read)"=w606:i16)
        n244 = case shown="\"Low (Assert High)\"" w620 {
          tunnel: [w645 w650] -> w626
          tunnel: [w644 w649] -> w625
          tunnel: w624 -> [w643 w648]
          tunnel: w623 -> [w642 w647]
          tunnel: w621 -> [w641 w646]
          frame "High (Assert Low)", Default {
            n245 = call <vilib>:"NI-845x SPI Script CS Low.vi"("error in (no error)"=w641, "chip select (0)"=w642, "spi script reference in"=w643) -> ("error out"=w645:errorcluster, "spi script reference out"=w644:T5)  [unwired: 7 in]
          }
          frame "Low (Assert High)" {
            n246 = call <vilib>:"NI-845x SPI Script CS High.vi"("error in (no error)"=w646, "chip select (0)"=w647, "spi script reference in"=w648) -> ("error out"=w650:errorcluster, "spi script reference out"=w649:T5)  [unwired: 7 in]
          }
        }
        n247 = Initialize Array(u16 255 ("element"), w606) -> (w610:u16[])
        n248 = To Unsigned Byte Integer(number=w608) -> (unsigned 8bit integer=w612:u8)
        n249 = To Unsigned Byte Integer(number=w607) -> (unsigned 8bit integer=w611:u8)
        n250 = Build Array (concatenate)(w612, w611, w610) -> (w605:u16[])
        n251 = call <vilib>:"NI-845x SPI Script Write Read.vi"("error in (no error)"=w626, "write data"=w605, "spi script reference in"=w625) -> ("error out"=w628:errorcluster, "script read index"=w618:u32, "spi script reference out"=w627:T5)  [unwired: 1 in, 5 out]
        n252 = Bundle By Name(cluster=w622, "script read index"=w618) -> (w619:T8)
        n253 = case shown="\"High (Assert Low)\", Default" w620 {
          tunnel: w628 -> [w635 w640]
          tunnel: w627 -> [w634 w639]
          tunnel: w623 -> [w633 w638]
          tunnel: [w632 w637] -> w615
          tunnel: [w631 w636] -> w614
          frame "High (Assert Low)", Default {
            n254 = call <vilib>:"NI-845x SPI Script CS High.vi"("error in (no error)"=w635, "chip select (0)"=w633, "spi script reference in"=w634) -> ("error out"=w632:errorcluster, "spi script reference out"=w631:T5)  [unwired: 7 in]
          }
          frame "Low (Assert High)" {
            n255 = call <vilib>:"NI-845x SPI Script CS Low.vi"("error in (no error)"=w640, "chip select (0)"=w638, "spi script reference in"=w639) -> ("error out"=w637:errorcluster, "spi script reference out"=w636:T5)  [unwired: 7 in]
          }
        }
        n256 = Multiply(x=u32 1 ("delay in microseconds (0)"), y=w606) -> (x*y=w617:u32)
        n257 = call-poly <vilib>:"NI-845x SPI Script Delay.vi"("error in (no error)"=w615, "delay in microseconds (0)"=w617, "spi script reference in"=w614) -> ("error out"=w613:errorcluster)  [unwired: 7 in, 1 out]
        n258 = call <vilib>:"Add State(s) to Queue__JKI_lib_State_Machine.vi"("State(s) in (\"\")"=w630) -> ("States Out"=w629:string)  [unwired: 14 in]
      }
      frame "NI845x: WRITE 93LC56BT" {
        # "For 93LC56BT the MSB is transmitted first (high endian)\nThe Microchip 93LC56BT CS idle state is LOW and asserted HIGH\nNote: the NI-8452 can only send 8-64 bits at a time. Make sure the INIT configures the device properly"
        n259 = Unbundle By Name(w661) -> ("CS/SS"=w653:u32, "Page Write Delay (ms)"=w655:u8, "SPI Script Reference"=w654:T5, "WRITE"=w656:u8, "EEPROM Program Data"=w657:string[][])
        n260 = for {
          tunnel: w658 -> [w683]
          tunnel: w654 -> [w682]
          tunnel: [w706] -> w652
          tunnel: w656 -> [w705]
          tunnel: w653 -> [w685]
          tunnel: [w684] -> w651
          tunnel: w655 -> [w679]
          tunnel: w657 -> [w672] mode=indexing
          # "Data"
          # "Address"
          # "Tcsl"
          n261 = call-poly <vilib>:"NI-845x SPI Script Delay.vi"("error in (no error)"=w683, "delay in milliseconds (0)"=w679, "spi script reference in"=w682) -> ("error out"=w680:errorcluster, "spi script reference out"=w681:T5)  [unwired: 7 out]
          n262 = Index Array(array=w672, index=0) -> (element=w675:string)
          n263 = Index Array(array=w672, index=1) -> (element=w678:string)
          n264 = call "Hex_String_to_Binary_String.vi"("bitness"=enum16{"8", "16", "32", "64"}."8", "Hexadecimal String"=w675) -> ("number"=w671:u64)  [unwired: 1 in, 2 out]
          n265 = call "Hex_String_to_Binary_String.vi"("bitness"=enum16{"8", "16", "32", "64"}."16", "Hexadecimal String"=w678) -> ("number"=w670:u64)  [unwired: 1 in, 2 out]
          n266 = To Unsigned Byte Integer(number=w671) -> (unsigned 8bit integer=w666:u8)
          n267 = To Unsigned Word Integer(number=w670) -> (unsigned 16bit integer=w669:u16)
          n268 = Split Number(x=w669) -> (hi(x)=w668:u8, lo(x)=w667:u8)
          n269 = To Unsigned Byte Integer(number=w705) -> (unsigned 8bit integer=w665:u8)
          n270 = call <vilib>:"NI-845x SPI Script CS High.vi"("error in (no error)"=w680, "chip select (0)"=w685, "spi script reference in"=w681) -> ("error out"=w696:errorcluster, "spi script reference out"=w697:T5)  [unwired: 7 in]
          n271 = Build Array(w665, w666, w668, w667) -> (w695:u8[])
          n272 = call <vilib>:"NI-845x SPI Script Write Read.vi"("error in (no error)"=w696, "write data"=w695, "spi script reference in"=w697) -> ("error out"=w704:errorcluster, "script read index"=w706:u32, "spi script reference out"=w703:T5)  [unwired: 1 in, 5 out]
          n273 = Array Subset(array=w695, index=2) -> (w664:u8[])  [unwired: 1 in]
          n274 = call <vilib>:"NI-845x SPI Script CS Low.vi"("error in (no error)"=w704, "chip select (0)"=w685, "spi script reference in"=w703) -> ("error out"=w702:errorcluster, "spi script reference out"=w701:T5)  [unwired: 7 in]
          n275 = local write "Data Bytes Written"(w664) -> ()
          n276 = call-poly <vilib>:"NI-845x SPI Script Delay.vi"("error in (no error)"=w702, "delay in microseconds (0)"=u16 1, "spi script reference in"=w701) -> ("error out"=w699:errorcluster, "spi script reference out"=w698:T5)  [unwired: 7 out]
          n277 = call <vilib>:"NI-845x SPI Script CS High.vi"("error in (no error)"=w699, "chip select (0)"=w685, "spi script reference in"=w698) -> ("error out"=w691:errorcluster, "spi script reference out"=w693:T5)  [unwired: 7 in]
          n278 = call-poly <vilib>:"NI-845x SPI Script Delay.vi"("error in (no error)"=w691, "delay in microseconds (0)"=u16 100, "spi script reference in"=w693) -> ("spi script reference out"=w690:T5)  [unwired: 8 out]
          n279 = call <vilib>:"NI-845x SPI Script CS Low.vi"("error in (no error)"=w691, "chip select (0)"=w685, "spi script reference in"=w690) -> ("error out"=w689:errorcluster, "spi script reference out"=w688:T5)  [unwired: 7 in]
          n280 = call <vilib>:"NI-845x SPI Script CS High.vi"("error in (no error)"=w689, "chip select (0)"=w685, "spi script reference in"=w688) -> ("error out"=w687:errorcluster, "spi script reference out"=w686:T5)  [unwired: 7 in]
          n281 = call <vilib>:"NI-845x SPI Script CS Low.vi"("error in (no error)"=w687, "chip select (0)"=w685, "spi script reference in"=w686) -> ("error out"=w684:errorcluster)  [unwired: 7 in, 1 out]
        }
        n282 = Bundle By Name(cluster=w661, "script read index"=w652) -> (w660:T8)
        n283 = call <vilib>:"Add State(s) to Queue__JKI_lib_State_Machine.vi"("State(s) in (\"\")"=w663, "State(s) at Back (\"\")"="UI: Display Message >>  [Alert!][WRITE Data Completed][10000]" ("State(s) in Front (\"\")")) -> ("States Out"=w662:string)  [unwired: 13 in]
      }
      frame "NI845x: READ 93C86" {
        # "For Microchip 93C86 the MSB is transmitted first (high endian)\nThe Microchip 93C86 CS idle state is LOW and asserted HIGH\nThis node needs the NI8452 model. NI845x only supports 8 bits"
        n284 = Unbundle By Name(w725) -> ("CS/SS"=w710:u32, "SPI Script Reference"=w716:T5, "READ"=w724:u8, "EEPROM Data Address"=w720:u16, "Number of Bytes (Read)"=w714:i16)
        n285 = Initialize Array(u16 255 ("element"), w714) -> (w707:u16[])
        n286 = call <vilib>:"NI-845x SPI Script CS High.vi"("error in (no error)"=w717, "chip select (0)"=w710, "spi script reference in"=w716) -> ("error out"=w715:errorcluster, "spi script reference out"=w726:T5)  [unwired: 7 in]
        n287 = Build Array (concatenate)(w724, w720, w707) -> (w721:u16[])
        n288 = call <vilib>:"NI-845x SPI Script Write Read.vi"("error in (no error)"=w715, "write data"=w721, "spi script reference in"=w726) -> ("error out"=w728:errorcluster, "script read index"=w722:u32, "spi script reference out"=w727:T5)  [unwired: 1 in, 5 out]
        n289 = call <vilib>:"NI-845x SPI Script CS Low.vi"("error in (no error)"=w728, "chip select (0)"=w710, "spi script reference in"=w727) -> ("error out"=w719:errorcluster, "spi script reference out"=w718:T5)  [unwired: 7 in]
        n290 = Bundle By Name(cluster=w725, "script read index"=w722) -> (w723:T8)
        n291 = call-poly <vilib>:"NI-845x SPI Script Delay.vi"("error in (no error)"=w719, "delay in milliseconds (0)"=u8 1, "spi script reference in"=w718) -> ("error out"=w713:errorcluster, "spi script reference out"=w711:T5)  [unwired: 7 in]
        n292 = call <vilib>:"NI-845x SPI Script CS High.vi"("error in (no error)"=w713, "chip select (0)"=w710, "spi script reference in"=w711) -> ("error out"=w712:errorcluster)  [unwired: 7 in, 1 out]
        n293 = call <vilib>:"Add State(s) to Queue__JKI_lib_State_Machine.vi"("State(s) in (\"\")"=w730) -> ("States Out"=w729:string)  [unwired: 14 in]
      }
      frame "NI845x: WRITE 93C86" {
        # "Index EEPROM\nProgram Data\nper row"
        # "For MC93C86 the MSB is transmitted first (high endian)\nThe Microchip 93C86 CS idle state is LOW and asserted HIGH\nNote: the NI-8452 can only send 8-64 bits at a time. Make sure the INIT configures the device properly"
        n294 = Unbundle By Name(w740) -> ("CS/SS"=w735:u32, "Page Write Delay (ms)"=w733:u8, "SPI Script Reference"=w739:T5, "WRITE"=w736:u8, "EEPROM Program Data"=w732:string[][])
        n295 = disable-structure shown="Disabled" {
          frame Disabled {
            (unwired) u8 0
            n296 = Reverse 1D Array() -> ()  [unwired: 1 in, 1 out]
            n297 = Build Array(u16 255 ("element"), u16 65535 ("element")) -> ()  [unwired: 1 in, 1 out]
          }
          frame Enabled {
          }
        }
        n298 = for {
          tunnel: w741 -> [w783]
          tunnel: w739 -> [w782]
          tunnel: [w780] -> w737
          tunnel: w736 -> [w766]
          tunnel: w735 -> [w778]
          tunnel: [w752] -> w734
          tunnel: w733 -> [w771]
          tunnel: w732 -> [w787] mode=indexing
          w750 = 0 items=["0 (First Edge)", "1 (Second Edge)"] ("clock phase (0)")
          w751 = 1 items=["0 (Idle Low)", "1 (Idle High)"] ("clock polarity (0)")
          w762 = 3 ("index")
          # "// force re-enable CLK by sending\ndummy data.\n// this satisfies the requirement\nto bring CS low before the next\nCLK rising edge."
          # "Data"
          # "Address"
          n299 = Index Array(array=w787, index=0) -> (element=w789:string)
          n300 = Index Array(array=w787, index=1) -> (element=w785:string)
          n301 = Number To Boolean Array(number=w766) -> (Boolean array=w765:bool[])
          n302 = Delete From Array(array=w765, length=w762, index=0) -> (deleted portion=w764:bool[])  [unwired: 1 out]
          n303 = call "Hex_String_to_Binary_String.vi"("bitness"=enum16{"8", "16", "32", "64"}."16", "Hexadecimal String"=w789) -> ("number"=w770:u64)  [unwired: 1 in, 2 out]
          n304 = call "Hex_String_to_Binary_String.vi"("bitness"=enum16{"8", "16", "32", "64"}."16", "Hexadecimal String"=w785) -> ("number"=w784:u64)  [unwired: 1 in, 2 out]
          n305 = Number To Boolean Array(number=w770) -> (Boolean array=w775:bool[])
          n306 = To Unsigned Word Integer(number=w784) -> (unsigned 16bit integer=w769:u16)
          n307 = Delete From Array(array=w775, length=10 ("index"), index=0) -> (deleted portion=w763:bool[])  [unwired: 1 out]
          n308 = Insert Into Array(array=w764, index=w762, new element=w763) -> (w761:bool[])
          n309 = Boolean Array To Number(Boolean array=w761) -> (number=w760:u32)
          n310 = To Unsigned Word Integer(number=w760) -> (unsigned 16bit integer=w759:u16)
          n311 = Split Number(x=w769) -> (hi(x)=w767:u8, lo(x)=w768:u8)
          n312 = Split Number(x=w759) -> (hi(x)=w756:u8, lo(x)=w757:u8)
          n313 = call <vilib>:"NI-845x SPI Script CS High.vi"("error in (no error)"=w783, "chip select (0)"=w778, "spi script reference in"=w782) -> ("error out"=w794:errorcluster, "spi script reference out"=w795:T5)  [unwired: 7 in]
          n314 = Build Array(w757, w756, w767, w768) -> (w772:u8[])
          n315 = call <vilib>:"NI-845x SPI Script Write Read.vi"("error in (no error)"=w794, "write data"=w772, "spi script reference in"=w795) -> ("error out"=w781:errorcluster, "script read index"=w780:u32, "spi script reference out"=w779:T5)  [unwired: 1 in, 5 out]
          n316 = Array Subset(array=w772, index=0) -> (w792:u8[])  [unwired: 1 in]
          n317 = call <vilib>:"NI-845x SPI Script CS Low.vi"("error in (no error)"=w781, "chip select (0)"=w778, "spi script reference in"=w779) -> ("error out"=w749:errorcluster, "spi script reference out"=w747:T5)  [unwired: 7 in]
          n318 = local write "Data Bytes Written"(w792) -> ()
          n319 = call <vilib>:"NI-845x SPI Script Clock Polarity Phase.vi"("error in (no error)"=w749, "clock phase (0)"=w750, "clock polarity (0)"=w751, "spi script reference in"=w747) -> ("error out"=w748:errorcluster, "spi script reference out"=w746:T5)  [unwired: 6 in]
          n320 = call-poly <vilib>:"NI-845x SPI Script Delay.vi"("error in (no error)"=w748, "delay in microseconds (0)"=u16 2, "spi script reference in"=w746) -> ("error out"=w755:errorcluster, "spi script reference out"=w754:T5)  [unwired: 7 in]
          n321 = call <vilib>:"NI-845x SPI Script CS High.vi"("error in (no error)"=w755, "chip select (0)"=w778, "spi script reference in"=w754) -> ("error out"=w777:errorcluster, "spi script reference out"=w776:T5)  [unwired: 7 in]
          n322 = call-poly <vilib>:"NI-845x SPI Script Delay.vi"("error in (no error)"=w777, "delay in milliseconds (0)"=w771, "spi script reference in"=w776) -> ("error out"=w752:errorcluster)  [unwired: 7 in, 1 out]
        }
        n323 = Bundle By Name(cluster=w740, "script read index"=w737) -> (w738:T8)
        n324 = call <vilib>:"Add State(s) to Queue__JKI_lib_State_Machine.vi"("State(s) in (\"\")"=w743, "State(s) at Back (\"\")"="UI: Display Message >>  [Alert!][WRITE Data Completed][10000]" ("State(s) in Front (\"\")")) -> ("States Out"=w742:string)  [unwired: 13 in]
      }
      frame "NI845x: READ [Generic]" {
        # "This is reserved for a generic EEPROM with data paging capability\n** Use this as a template for other EEPROM device types **\nSEE DEVICE DATA SHEET FOR TIMING INFORMATION"
        n325 = Unbundle By Name(w808) -> ("CS/SS"=w809:u32, "CS Idle Level"=w803:enum16{"Low (Assert High)", "High (Assert Low)"}, "SPI Script Reference"=w810:T5, "EEPROM Device Type"=w800:T2, "READ"=w804:u8, "Data Address Endianness"=w805:bool, "EEPROM Data Address"=w798:u16, "Number of Bytes (Read)"=w799:i16, "Target Page Size (bytes)"=w797:i32)
        n326 = call "CreateWriteCluster.vi"("Page Size in Bytes"=w797, "EEPROM Starting Address"=w798, "Number of Bytes to Write"=w799) -> ("Array of Write Cluster Information"=w796:T10)  [unwired: 1 in]
        n327 = for {
          tunnel: w810 -> [w831]
          tunnel: w809 -> [w830]
          tunnel: w807 -> [w829]
          tunnel: [w828] -> w806
          tunnel: w805 -> [w827]
          tunnel: w804 -> [w826]
          tunnel: w803 -> [w825]
          tunnel: [w824] -> w801
          tunnel: w800 -> [w817]
          tunnel: w796 -> [w816] mode=indexing
          n328 = case shown="\"Low (Assert High)\"" w825 {
            tunnel: [w871 w876] -> w833
            tunnel: [w870 w875] -> w832
            tunnel: w831 -> [w869 w874]
            tunnel: w830 -> [w868 w873]
            tunnel: w829 -> [w867 w872]
            frame "High (Assert Low)", Default {
              n329 = call <vilib>:"NI-845x SPI Script CS Low.vi"("error in (no error)"=w867, "chip select (0)"=w868, "spi script reference in"=w869) -> ("error out"=w871:errorcluster, "spi script reference out"=w870:T5)  [unwired: 7 in]
            }
            frame "Low (Assert High)" {
              n330 = call <vilib>:"NI-845x SPI Script CS High.vi"("error in (no error)"=w872, "chip select (0)"=w873, "spi script reference in"=w874) -> ("error out"=w876:errorcluster, "spi script reference out"=w875:T5)  [unwired: 7 in]
            }
          }
          n331 = Unbundle By Name(w816) -> ("EEPROM Address"=w813:u16, "Data Index"=w814:u32, "Length"=w815:u32)
          n332 = Select(t=i16 0, s=w827, f=i16 -8) -> (s? t:f=w820:i16)
          n333 = Rotate(1:w813, 2:w820) -> (0:w819:u16)
          n334 = Initialize Array(w814, w815) -> (w818:u32[])
          n335 = case shown="\"Microchip LC56BT\", Default" w817 {
            tunnel: w819 -> [w839 w857]
            tunnel: [w837 w858] -> w823
            tunnel: w826 -> [w838 w852]
            tunnel: w827 -> [_ w853]
            tunnel: w818 -> [w836 w842]
            tunnel: w813 -> [_ w843]
            frame "Microchip 93C86" {
              n336 = Split Number(x=w839) -> (hi(x)=w841:u8, lo(x)=w840:u8)
              n337 = Build Array (concatenate)(w838, w841, w840, w836) -> (w837:u32[])
            }
            frame "Microchip LC56BT", Default {
              n338 = Number To Boolean Array(number=w843) -> (Boolean array=w845:bool[])
              n339 = Number To Boolean Array(number=w852) -> (Boolean array=w851:bool[])
              n340 = Split Number(x=w857) -> (hi(x)=w855:u8, lo(x)=w856:u8)
              n341 = Index Array(array=w845, index=8) -> (element=w844:bool)
              n342 = Replace Array Subset(array=w851, new element=w844, index=3) -> (w849:bool[])
              n343 = Select(t=w856, s=w853, f=w855) -> (s? t:f=w854:u8)
              n344 = Boolean Array To Number(Boolean array=w849) -> (number=w848:u32)
              n345 = To Unsigned Byte Integer(number=w848) -> (unsigned 8bit integer=w847:u8)
              n346 = Build Array (concatenate)(w847, w854, w842) -> (w858:u32[])
            }
          }
          n347 = call <vilib>:"NI-845x SPI Script Write Read.vi"("error in (no error)"=w833, "write data"=w823, "spi script reference in"=w832) -> ("error out"=w835:errorcluster, "script read index"=w824:u32, "spi script reference out"=w834:T5)  [unwired: 1 in, 5 out]
          n348 = case shown="\"Low (Assert High)\"" w825 {
            tunnel: w835 -> [w862 w866]
            tunnel: w834 -> [w861 w865]
            tunnel: w830 -> [w860 w864]
            tunnel: [w859 w863] -> w828
            frame "High (Assert Low)", Default {
              n349 = call <vilib>:"NI-845x SPI Script CS High.vi"("error in (no error)"=w862, "chip select (0)"=w860, "spi script reference in"=w861) -> ("error out"=w859:errorcluster)  [unwired: 7 in, 1 out]
            }
            frame "Low (Assert High)" {
              n350 = call <vilib>:"NI-845x SPI Script CS Low.vi"("error in (no error)"=w866, "chip select (0)"=w864, "spi script reference in"=w865) -> ("error out"=w863:errorcluster)  [unwired: 7 in, 1 out]
            }
          }
        }
        n351 = Bundle By Name(cluster=w808, "script read index"=w801) -> (w802:T8)
        n352 = call <vilib>:"Add State(s) to Queue__JKI_lib_State_Machine.vi"("State(s) in (\"\")"=w812) -> ("States Out"=w811:string)  [unwired: 14 in]
      }
      frame "NI845x: WRITE [Generic]" {
        # "This is reserved for a generic EEPROM with data paging capability\n** Use this as a template for other EEPROM device types **\nSEE DEVICE DATA SHEET FOR TIMING INFORMATION"
        n353 = Unbundle By Name(w893) -> ("CS/SS"=w884:u32, "CS Idle Level"=w885:enum16{"Low (Assert High)", "High (Assert Low)"}, "EEPROM Device Type"=w883:T2, "Page Write Delay (ms)"=w891:u8, "SPI Script Reference"=w892:T5, "Data Address Endianness"=w890:bool, "WRITE"=w887:u8, "EEPROM Data Address"=w882:u16, "Number of Bytes (Read)"=w879:i16, "Target Page Size (bytes)"=w881:i32, "Bit Pattern (Write All)"=w878:T4)
        n354 = for {
          N: w879 -> [_]
          tunnel: w878 -> [w898]
          tunnel: [w897] -> w877 mode=indexing
          n355 = case shown="\"0xAA (0b10101010)\"" w898 {
            tunnel: [u8 255 u8 0 u8 170 u8 85] -> w897
            frame "All ONES", Default {
            }
            frame "All ZEROES" {
            }
            frame "0xAA (0b10101010)" {
            }
            frame "0x55 (0b01010101)" {
            }
          }
        }
        n356 = call "CreateWriteCluster.vi"("Page Size in Bytes"=w881, "EEPROM Starting Address"=w882, "Number of Bytes to Write"=w879) -> ("Array of Write Cluster Information"=w880:T10)  [unwired: 1 in]
        n357 = for {
          tunnel: w894 -> [w912]
          tunnel: w892 -> [w911]
          tunnel: w891 -> [_]
          tunnel: w883 -> [w933]
          tunnel: w890 -> [w932]
          tunnel: [w931] -> w888
          tunnel: w887 -> [w930]
          tunnel: w884 -> [w923]
          tunnel: w885 -> [w922]
          tunnel: [w924] -> w886
          tunnel: w885 -> [w910]
          tunnel: w884 -> [w909]
          tunnel: w880 -> [w908] mode=indexing
          tunnel: w877 -> [w905]
          w914 = 2 ("index")
          # "Tcsl"
          n358 = Select(t=i16 0, s=w932, f=i16 -8) -> (s? t:f=w919:i16)
          n359 = Unbundle By Name(w908) -> ("EEPROM Address"=w907:u16, "Data Index"=w904:u32, "Length"=w906:u32)
          n360 = Rotate(1:w907, 2:w919) -> (0:w916:u16)
          n361 = Array Subset(array=w905, index=w904, length=w906) -> (w903:u8[])
          n362 = case shown="\"Microchip LC56BT\", Default" w933 {
            tunnel: [w945 w966] -> w915
            tunnel: w916 -> [w946 w965]
            tunnel: w930 -> [w947 w955]
            tunnel: w932 -> [_ w963]
            tunnel: w903 -> [w944 w951]
            tunnel: w907 -> [_ w950]
            frame "Microchip 93C86" {
              n363 = Split Number(x=w946) -> (hi(x)=w948:u8, lo(x)=w949:u8)
              n364 = Build Array (concatenate)(w947, w948, w949, w944) -> (w945:u8[])
            }
            frame "Microchip LC56BT", Default {
              n365 = Number To Boolean Array(number=w950) -> (Boolean array=w954:bool[])
              n366 = Split Number(x=w965) -> (hi(x)=w964:u8, lo(x)=w962:u8)
              n367 = Number To Boolean Array(number=w955) -> (Boolean array=w960:bool[])
              n368 = Index Array(array=w954, index=8) -> (element=w952:bool)
              n369 = Replace Array Subset(array=w960, new element=w952, index=3) -> (w958:bool[])
              n370 = Boolean Array To Number(Boolean array=w958) -> (number=w957:u32)
              n371 = Select(t=w962, s=w963, f=w964) -> (s? t:f=w961:u8)
              n372 = To Unsigned Byte Integer(number=w957) -> (unsigned 8bit integer=w956:u8)
              n373 = Build Array (concatenate)(w956, w961, w951) -> (w966:u8[])
            }
          }
          n374 = case shown="\"Low (Assert High)\"" w910 {
            tunnel: [w938 w943] -> w918
            tunnel: [w937 w942] -> w917
            tunnel: w912 -> [w936 w941]
            tunnel: w911 -> [w935 w940]
            tunnel: w909 -> [w934 w939]
            frame "High (Assert Low)" {
              n375 = call <vilib>:"NI-845x SPI Script CS Low.vi"("error in (no error)"=w936, "chip select (0)"=w934, "spi script reference in"=w935) -> ("error out"=w937:errorcluster, "spi script reference out"=w938:T5)  [unwired: 7 in]
            }
            frame "Low (Assert High)" {
              n376 = call <vilib>:"NI-845x SPI Script CS High.vi"("error in (no error)"=w941, "chip select (0)"=w939, "spi script reference in"=w940) -> ("error out"=w942:errorcluster, "spi script reference out"=w943:T5)  [unwired: 7 in]
            }
          }
          n377 = call <vilib>:"NI-845x SPI Script Write Read.vi"("error in (no error)"=w917, "write data"=w915, "spi script reference in"=w918) -> ("error out"=w929:errorcluster, "script read index"=w931:u32, "spi script reference out"=w928:T5)  [unwired: 1 in, 5 out]
          n378 = Array Subset(array=w915, index=w914, length=w914) -> (w913:u8[])
          n379 = case shown="\"Low (Assert High)\"" w922 {
            tunnel: [w971 w976] -> w927
            tunnel: [w970 w975] -> w926
            tunnel: w929 -> [w969 w974]
            tunnel: w928 -> [w968 w973]
            tunnel: w923 -> [w967 w972]
            frame "High (Assert Low)" {
              n380 = call <vilib>:"NI-845x SPI Script CS High.vi"("error in (no error)"=w969, "chip select (0)"=w967, "spi script reference in"=w968) -> ("error out"=w971:errorcluster, "spi script reference out"=w970:T5)  [unwired: 7 in]
            }
            frame "Low (Assert High)" {
              n381 = call <vilib>:"NI-845x SPI Script CS Low.vi"("error in (no error)"=w974, "chip select (0)"=w972, "spi script reference in"=w973) -> ("error out"=w976:errorcluster, "spi script reference out"=w975:T5)  [unwired: 7 in]
            }
          }
          n382 = local write "Data Bytes Written"(w913) -> ()
          n383 = call-poly <vilib>:"NI-845x SPI Script Delay.vi"("error in (no error)"=w927, "delay in microseconds (0)"=u16 1, "spi script reference in"=w926) -> ("error out"=w924:errorcluster)  [unwired: 8 out]
        }
        n384 = Bundle By Name(cluster=w893, "script read index"=w888) -> (w889:T8)
        n385 = call <vilib>:"Add State(s) to Queue__JKI_lib_State_Machine.vi"("State(s) in (\"\")"=w896) -> ("States Out"=w895:string)  [unwired: 14 in]
      }
      frame "NI845x: EWDS" {
        w978 = 0 items=["0 (First Edge)", "1 (Second Edge)"] ("clock phase (0)")
        w979 = 0 items=["0 (Idle Low)", "1 (Idle High)"] ("clock polarity (0)")
        # "1. Send SB & EWDS Opcode\n2. A dummy address byte\n3. A dummy data byte"
        n386 = Unbundle By Name(w991) -> ("EWDS"=w989:u8, "EEPROM Device Type"=w977:T2, "SPI Script Reference"=w982:T5, "CS/SS"=w985:u32, "CS Idle Level"=w986:enum16{"Low (Assert High)", "High (Assert Low)"})
        n387 = call <vilib>:"NI-845x SPI Script Clock Polarity Phase.vi"("error in (no error)"=w984, "clock phase (0)"=w978, "clock polarity (0)"=w979, "spi script reference in"=w982) -> ("error out"=w983:errorcluster, "spi script reference out"=w981:T5)  [unwired: 6 in]
        n388 = case shown="\"Low (Assert High)\"" w986 {
          tunnel: w981 -> [w1006 w1011]
          tunnel: w983 -> [w1005 w1010]
          tunnel: [w1004 w1009] -> _
          tunnel: w985 -> [w1003 w1008]
          tunnel: [w1002 w1007] -> w988
          frame "High (Assert Low)" {
            n389 = call <vilib>:"NI-845x SPI Script CS High.vi"("error in (no error)"=w1005, "chip select (0)"=w1003, "spi script reference in"=w1006) -> ("error out"=w1004:errorcluster, "spi script reference out"=w1002:T5)  [unwired: 7 in]
          }
          frame "Low (Assert High)" {
            n390 = call <vilib>:"NI-845x SPI Script CS Low.vi"("error in (no error)"=w1010, "chip select (0)"=w1008, "spi script reference in"=w1011) -> ("error out"=w1009:errorcluster, "spi script reference out"=w1007:T5)  [unwired: 7 in]
          }
        }
        n391 = case shown="\"Microchip 93C86\"" w977 {
          tunnel: [u8 0 u8 0 u16 0] -> w996
          frame "Microchip LC56BT", Default {
          }
          frame "Generic EEPROM" {
          }
          frame "Microchip 93C86" {
          }
        }
        n392 = case shown="\"Low (Assert High)\"" w986 {
          tunnel: w983 -> [w1024 w1029]
          tunnel: w988 -> [w1023 w1028]
          tunnel: [w1022 w1027] -> w990
          tunnel: w985 -> [w1021 w1026]
          tunnel: [w1020 w1025] -> w987
          frame "High (Assert Low)" {
            n393 = call <vilib>:"NI-845x SPI Script CS Low.vi"("error in (no error)"=w1024, "chip select (0)"=w1021, "spi script reference in"=w1023) -> ("error out"=w1020:errorcluster, "spi script reference out"=w1022:T5)  [unwired: 7 in]
          }
          frame "Low (Assert High)" {
            n394 = call <vilib>:"NI-845x SPI Script CS High.vi"("error in (no error)"=w1029, "chip select (0)"=w1026, "spi script reference in"=w1028) -> ("error out"=w1025:errorcluster, "spi script reference out"=w1027:T5)  [unwired: 7 in]
          }
        }
        n395 = To Unsigned Byte Integer(number=w989) -> (unsigned 8bit integer=w980:u8)
        n396 = Build Array(w980, w996, w996) -> (w995:u16[])
        n397 = call <vilib>:"NI-845x SPI Script Write Read.vi"("error in (no error)"=w987, "write data"=w995, "spi script reference in"=w990) -> ("error out"=w993:errorcluster, "spi script reference out"=w994:T5)  [unwired: 1 in, 6 out]
        n398 = case shown="\"Low (Assert High)\"" w986 {
          tunnel: w994 -> [w1015 w1019]
          tunnel: w993 -> [w1014 w1018]
          tunnel: [w1013 w1017] -> w992
          tunnel: w985 -> [w1012 w1016]
          frame "High (Assert Low)" {
            n399 = call <vilib>:"NI-845x SPI Script CS High.vi"("error in (no error)"=w1014, "chip select (0)"=w1012, "spi script reference in"=w1015) -> ("error out"=w1013:errorcluster)  [unwired: 7 in, 1 out]
          }
          frame "Low (Assert High)" {
            n400 = call <vilib>:"NI-845x SPI Script CS Low.vi"("error in (no error)"=w1018, "chip select (0)"=w1016, "spi script reference in"=w1019) -> ("error out"=w1017:errorcluster)  [unwired: 7 in, 1 out]
          }
        }
        n401 = call <vilib>:"Add State(s) to Queue__JKI_lib_State_Machine.vi"("State(s) in (\"\")"=w998) -> ("States Out"=w997:string)  [unwired: 14 in]
      }
      frame "NI845x: Erase ALL" {
        # "Then assert the CS line\nto start the ERASE ALL\ncycle. The ERASE ALL\ncycle is self-timed. \nNo need to CLK"
        # "Delay for Tcsl"
        # "1. Send SB & ERAL Opcode\n2. A dummy address byte\n3. A dummy data byte"
        n402 = Unbundle By Name(w1048) -> ("EEPROM Device Type"=w1036:T2, "ERAL"=w1045:u8, "SPI Script Reference"=w1047:T5, "CS/SS"=w1038:u32, "Page Write Delay (ms)"=w1030:u8)
        n403 = case shown="\"Microchip LC56BT\", Default" w1036 {
          tunnel: [w1058 w1063] -> w1052
          tunnel: w1045 -> [w1057 w1062]
          frame "Microchip LC56BT", Default {
            w1056 = u8 0 ("element")
            # "16-bit Data & 8-bit Address"
            n404 = To Unsigned Byte Integer(number=w1057) -> (unsigned 8bit integer=w1055:u8)
            n405 = Build Array(w1055, w1056, w1056) -> (w1058:u8[])
          }
          frame "Microchip 93C86" {
            # "16-bit Data & Address"
            n406 = To Unsigned Byte Integer(number=w1062) -> (unsigned 8bit integer=w1061:u8)
            n407 = Build Array(w1061, u8 0 ("element"), u16 0 ("element")) -> (w1063:u16[])
          }
        }
        n408 = call <vilib>:"NI-845x SPI Script CS High.vi"("error in (no error)"=w1049, "chip select (0)"=w1038, "spi script reference in"=w1047) -> ("error out"=w1041:errorcluster, "spi script reference out"=w1046:T5)  [unwired: 7 in]
        n409 = call <vilib>:"NI-845x SPI Script Write Read.vi"("error in (no error)"=w1041, "write data"=w1052, "spi script reference in"=w1046) -> ("error out"=w1050:errorcluster, "script read index"=w1034:u32, "spi script reference out"=w1051:T5)  [unwired: 1 in, 5 out]
        n410 = Bundle By Name(cluster=w1048, "script read index"=w1034) -> (w1035:T8)
        n411 = call <vilib>:"NI-845x SPI Script CS Low.vi"("error in (no error)"=w1050, "chip select (0)"=w1038, "spi script reference in"=w1051) -> ("error out"=w1044:errorcluster, "spi script reference out"=w1043:T5)  [unwired: 7 in]
        n412 = call-poly <vilib>:"NI-845x SPI Script Delay.vi"("error in (no error)"=w1044, "delay in microseconds (0)"=u16 1, "spi script reference in"=w1043) -> ("error out"=w1040:errorcluster, "spi script reference out"=w1039:T5)  [unwired: 7 in]
        n413 = call <vilib>:"NI-845x SPI Script CS High.vi"("error in (no error)"=w1040, "chip select (0)"=w1038, "spi script reference in"=w1039) -> ("error out"=w1033:errorcluster, "spi script reference out"=w1032:T5)  [unwired: 7 in]
        n414 = call <vilib>:"Add State(s) to Queue__JKI_lib_State_Machine.vi"("State(s) in Front (\"\")"="UI: Display Message >>  [Alert!][ERASE ALL Completed][10000]" ("State(s) in Front (\"\")"), "State(s) in (\"\")"=w1054) -> ("States Out"=w1053:string)  [unwired: 13 in]
        n415 = call-poly <vilib>:"NI-845x SPI Script Delay.vi"("error in (no error)"=w1033, "delay in milliseconds (0)"=w1030, "spi script reference in"=w1032) -> ("error out"=w1031:errorcluster)  [unwired: 7 in, 1 out]
      }
      frame "NI845x: Write ALL" {
        # "Delay for Tcsl"
        # "1. Send SB & WRAL opcode.\n2. A dummy address byte.\n3. Desired data pattern to write."
        n416 = Unbundle By Name(w1091) -> ("Bit Pattern (Write All)"=w1074:T4, "WRAL"=w1089:u8, "EEPROM Device Type"=w1064:T2, "SPI Script Reference"=w1075:T5, "CS/SS"=w1077:u32, "Page Write Delay (ms)"=w1078:u8)
        n417 = case shown="\"0x55 (0b01010101)\"" w1074 {
          tunnel: [u16 65535 u16 0 u16 43690 u16 61166 u16 21845] -> w1073
          frame "All ONES", Default {
          }
          frame "All ZEROES" {
          }
          frame "0xAA (0b10101010)" {
          }
          frame "0xEE (0b11101110)" {
          }
          frame "0x55 (0b01010101)" {
          }
        }
        n418 = case shown="\"Microchip 93C86\", Default" w1064 {
          tunnel: [w1115 w1129] -> w1094
          tunnel: w1089 -> [w1114 w1128]
          tunnel: w1073 -> [w1113 w1124]
          frame "Microchip LC56BT" {
            # "16-bit Data & 8-bit Address"
            n419 = To Unsigned Byte Integer(number=w1114) -> (unsigned 8bit integer=w1111:u8)
            n420 = Split Number(x=w1113) -> (hi(x)=w1110:u8, lo(x)=w1112:u8)
            n421 = Build Array(w1111, u8 0 ("element"), w1110, w1112) -> (w1115:u8[])
          }
          frame "Microchip 93C86", Default {
            # "10-bit Address & 16-bit Data"
            n422 = Number To Boolean Array(number=w1128) -> (Boolean array=w1127:bool[])
            n423 = Number To Boolean Array(number=w1124) -> (Boolean array=w1123:bool[])
            n424 = Delete From Array(array=w1127, length=5, index=0) -> (deleted portion=w1120:bool[])  [unwired: 1 out]
            n425 = Reverse 1D Array(array=w1123) -> (reversed array=w1122:bool[])
            n426 = Boolean Array To Number(Boolean array=w1120) -> (number=w1119:u32)
            n427 = Boolean Array To Number(Boolean array=w1122) -> (number=w1121:u32)
            n428 = To Unsigned Word Integer(number=w1121) -> (unsigned 16bit integer=w1117:u16)
            n429 = To Unsigned Byte Integer(number=w1119) -> (unsigned 8bit integer=w1116:u8)
            n430 = Build Array(w1116, u16 0 ("element"), w1117, w1117) -> (w1129:u16[])
          }
        }
        n431 = call <vilib>:"NI-845x SPI Script CS High.vi"("error in (no error)"=w1076, "chip select (0)"=w1077, "spi script reference in"=w1075) -> ("error out"=w1087:errorcluster, "spi script reference out"=w1090:T5)  [unwired: 7 in]
        n432 = call <vilib>:"NI-845x SPI Script Write Read.vi"("error in (no error)"=w1087, "write data"=w1094, "spi script reference in"=w1090) -> ("error out"=w1092:errorcluster, "script read index"=w1082:u32, "spi script reference out"=w1093:T5)  [unwired: 1 in, 5 out]
        n433 = Bundle By Name(cluster=w1091, "script read index"=w1082) -> (w1083:T8)
        n434 = call <vilib>:"NI-845x SPI Script CS Low.vi"("error in (no error)"=w1092, "chip select (0)"=w1077, "spi script reference in"=w1093) -> ("error out"=w1069:errorcluster, "spi script reference out"=w1068:T5)  [unwired: 7 in]
        n435 = Build Array(u8 5, u16 0 ("element"), u16 255 ("element")) -> (w1067:u16[])
        n436 = disable-structure shown="Disabled" {
          disable-tunnel: w1069 -> [w1101 w1103]
          disable-tunnel: w1068 -> [w1100 w1102]
          disable-tunnel: w1067 -> [w1099 _]
          disable-tunnel: [w1098 w1103] -> w1066
          disable-tunnel: [w1097 w1102] -> w1065
          frame Disabled {
            n437 = call <vilib>:"NI-845x SPI Script Write Read.vi"("error in (no error)"=w1101, "write data"=w1099, "spi script reference in"=w1100) -> ("error out"=w1098:errorcluster, "spi script reference out"=w1097:T5)  [unwired: 1 in, 6 out]
          }
          frame Enabled {
          }
        }
        n438 = call-poly <vilib>:"NI-845x SPI Script Delay.vi"("error in (no error)"=w1066, "delay in microseconds (0)"=u16 2, "spi script reference in"=w1065) -> ("error out"=w1086:errorcluster, "spi script reference out"=w1085:T5)  [unwired: 7 in]
        n439 = call <vilib>:"NI-845x SPI Script CS High.vi"("error in (no error)"=w1086, "chip select (0)"=w1077, "spi script reference in"=w1085) -> ("error out"=w1080:errorcluster, "spi script reference out"=w1081:T5)  [unwired: 7 in]
        n440 = call <vilib>:"Add State(s) to Queue__JKI_lib_State_Machine.vi"("State(s) in Front (\"\")"="UI: Display Message >>  [Alert!][WRITE ALL Completed][10000]" ("State(s) in Front (\"\")"), "State(s) in (\"\")"=w1096) -> ("States Out"=w1095:string)  [unwired: 13 in]
        n441 = call-poly <vilib>:"NI-845x SPI Script Delay.vi"("error in (no error)"=w1080, "delay in milliseconds (0)"=w1078, "spi script reference in"=w1081) -> ("error out"=w1079:errorcluster)  [unwired: 7 in, 1 out]
      }
      frame "NI845x: RUN Script - Read Data - Close Device" {
        # "Close SPI bus, Run Script, Read the Data Array from Device, Close the reference to Device"
        n442 = Unbundle By Name(w1141) -> ("EEPROM Device Type"=w1132:T2, "script read index"=w1135:u32, "NI845x Device ID"=w1134:T3, "SPI Script Reference"=w1142:T5)
        n443 = case shown="\"Microchip 93C86\", Default" w1132 {
          tunnel: [3 ("index") 2 ("index")] -> w1133
          frame "Microchip 93C86", Default {
          }
          frame "Microchip LC56BT" {
          }
        }
        n444 = call <vilib>:"NI-845x SPI Script Disable SPI.vi"("error in (no error)"=w1144, "spi script reference in"=w1142) -> ("error out"=w1145:errorcluster, "spi script reference out"=w1146:T5)  [unwired: 8 out]
        n445 = call <vilib>:"NI-845x SPI Run Script.vi"("error in (no error)"=w1145, "device reference in"=w1134, "spi script reference in"=w1146) -> ("error out"=w1139:errorcluster, "spi script reference out"=w1140:T5)  [unwired: 1 in, 6 out]
        n446 = call <vilib>:"NI-845x SPI Extract Script Read Data.vi"("error in (no error)"=w1139, "script read index"=w1135, "spi script reference in"=w1140) -> ("error out"=w1138:errorcluster, "read data"=w1136:u8[], "spi script reference out"=w1137:T5)  [unwired: 6 out]
        n447 = Array Subset(array=w1136, index=w1133) -> (w1130:u8[])  [unwired: 1 in]
        n448 = call-poly <vilib>:"NI-845x Close Reference.vi"("error in (no error)"=w1138, "spi script reference"=w1137) -> ("error out"=w1143:errorcluster)  [unwired: 9 out]
        n449 = local write "Read Data"(w1130) -> ()
        n450 = Bundle By Name(cluster=w1141, "Read Data"=w1130) -> (w1131:T8)
        n451 = call <vilib>:"Add State(s) to Queue__JKI_lib_State_Machine.vi"("State(s) in (\"\")"=w1148) -> ("States Out"=w1147:string)  [unwired: 14 in]
      }
      frame "NI845x: Run Script - Close SPI - Close Device" {
        n452 = Unbundle By Name(w1154) -> ("NI845x Device ID"=w1151:T3, "SPI Script Reference"=w1155:T5)
        n453 = call <vilib>:"NI-845x SPI Script Disable SPI.vi"("error in (no error)"=w1157, "spi script reference in"=w1155) -> ("error out"=w1158:errorcluster, "spi script reference out"=w1159:T5)  [unwired: 8 out]
        n454 = call <vilib>:"NI-845x SPI Run Script.vi"("error in (no error)"=w1158, "device reference in"=w1151, "spi script reference in"=w1159) -> ("error out"=w1152:errorcluster, "spi script reference out"=w1153:T5)  [unwired: 1 in, 6 out]
        n455 = call-poly <vilib>:"NI-845x Close Reference.vi"("error in (no error)"=w1152, "spi script reference"=w1153) -> ("error out"=w1156:errorcluster)  [unwired: 9 out]
        n456 = call <vilib>:"Add State(s) to Queue__JKI_lib_State_Machine.vi"("State(s) in (\"\")"=w1161) -> ("States Out"=w1160:string)  [unwired: 14 in]
      }
    }
  }
